vi "RG TAS v4.vi"() -> ()   [LabVIEW 2015]
uses:
  <vilib>/Analysis/2dsp.llb/Decimate (single shot, DBL).vi
  <vilib>/DAQmx/read.llb/DAQmx Read (Analog Wfm 1Chan NSamp).vi
  Chaz TAS - DR/Sub VIs/Mono/global_Test.vi
  <vilib>/Instr/_visa.llb/VISA Configure Serial Port (Instr).vi
  Sub VIs/global tas.vi
  <vilib>/DAQmx/miscellaneous.llb/DAQmx Fill In Error Info.vi
  <vilib>/Utility/file.llb/Write To Spreadsheet File (DBL).vi
  <vilib>/Waveform/WDTOps.llb/WDT Index Channel DBL.vi
  Program Files/National Instruments/LabVIEW 2014/instr.lib/Tektronix DPO MSO 2000 4000 Series/Tektronix DPO MSO 2000 4000 Series.lvlib
  <vilib>/Analysis/NI_AALPro.lvlib
panel:
  out "DAQ Loop":i32
  out "Scope Error Counter":i32
  out "Scope time axis":dbl[](array[numeric])
  in  "Stop acquisition":bool
  out "Grating":i32
  in  "2b - Spectrum":bool
  in  "2a - Kinetic":bool
  in  "Stop":bool
  out "Btrace Readout Counter":i32=2
  in  "Stop Btrace Measurement":bool
  out "Readout Counter":i32=2
  in  "Stop Measurement":bool
  in  "Calculate Output Method":T1(ring)
  in  "Parameters":T2(tab)
  in  "Shutter flow control":u16(ring) items=["None"=0, "XON/XOFF"=1, "RTS/CTS"=2, "DTR/DSR"=4]
  in  "Shutter stop bits":u16(ring)=10 items=["1.0"=10, "1.5"=15, "2.0"=20]
  in  "Shutter parity":u16(ring) items=["None", "Odd", "Even", "Mark", "Space"]
  in  "Shutter data bits":u16=8 min=5 max=8 step=1
  in  "Shutter VISA resource name":refnum<visa-resource-name>="COM1"
  in  "Shutter baud rate":u32=9600
  in  "Shutter open string":string="+100 10\n"
  in  "1 - Move Shutter":bool
  in  "3 - Move mono":bool
  out "Current wavelength (Oriel)":dbl format="%#_13g"
  in  "Monochromator Type":bool
  out "Start Wavelength":dbl min=0.0 format="%.3f"
  out "End Wavelength":dbl=100.0 min=0.0 format="%.3f"
  out "Interval Wavelength":dbl=10.0 min=0.0 format="%.3f"
  out "Current Wavelength (PTI)":dbl=300.0 min=300.0 max=2000.0 step=1.0
  in  "Is IR":bool caption="Grating"
  in  "Mono VISA name":refnum<visa-resource-name>
  in  "Mono 2 VISA name":refnum<visa-resource-name>
  out "DAQ dt":dbl=5e-06
  in  "DAQ End Time":dbl=0.05
  in  "DAQ rate":i32=1250000
  in  "DAQ Trigger Level (V)":dbl=0.2
  out "DAQ Number of Samples":dbl=10000.0
  in  "DAQ average number of points":dbl=1.0
  out "DAQ final number of points":dbl
  in  "DAQ Input Channel":tag="Dev1/ai0"
  in  "100% Reflectance Standard (V)":dbl=1.0
  in  "DAQ Card":enum16{"USB-6211", "USB-6251"}(ring)=enum."USB-6251"
  in  "DAQ Input Config":i32(ring)=10106 items=["default"=-1, "RSE"=10083, "NRSE"=10078, "Differential"=10106, "Pseudodifferential"=12529]
  in  "Record Length":u32(ring)=10 items=["1000 points"=1, "10k points"=10, "100k points"=100, "1M points"=1000, "5M points"=5000, "10M points"=10000]
  in  "Acquisition Type":u16(ring)=2 items=["Sample", "Peak Detect", "Hi Res", "Envelope", "Average"]
  in  "Scope average\nnumber of points":dbl=1.0
  in  "Averages on scope":i32=1
  in  "Using TDS Scope?":bool
  in  "CH2 Impedance":u16(ring) items=["1M", "75", "50"]
  in  "CH1 Impedance":u16(ring)=2 items=["1M", "75", "50"]
  in  "Scope VISA resource name":refnum<visa-resource-name>="USB0::0x0699::0x0410::C022077::INSTR"
  in  "Scope Timeout (ms)":u32=30000
  in  "Channel TAS (0: Channel 1)":u16(ring) caption="Channel TAS" items=["Channel 1", "Channel 2", "Channel 3", "Channel 4", "Math", "Reference A", "Reference B", "Reference C", "Reference D"]
  in  "Channel TPC (0: Channel 1)":u16(ring)=1 caption="Channel TPC" items=["Channel 1", "Channel 2", "Channel 3", "Channel 4", "Math", "Reference A", "Reference B", "Reference C", "Reference D"]
  in  "Scope Timebase":dbl=0.0004 format="%^#_3e"
  in  "Trigger Source":u16(ring)=1 items=["Channel 1", "Channel 2", "Channel 3", "Channel 4", "AC Line", "Aux", "Digital Channel 0", "Digital Channel 1", "Digital Channel 2", "Digital Channel 3", "Digital Channel 4", "Digital Channel 5", "Digital Channel 6", "Digital Channel 7", "Digital Channel 8", "Digital Channel 9", "Digital Channel 10", "Digital Channel 11", "Digital Channel 12", "Digital Channel 13", "Digital Channel 14", "Digital Channel 15", "RF"]
  out "Final number of\nscope points":dbl=10000.0
  in  "Vertical Coupling TAS (1: DC)":u16(ring)=1 caption="Vertical Coupling TAS" items=["AC", "DC", "Ground"]
  in  "Probe Attenuation TAS (10.0)":dbl=1.0 caption="Probe Attenuation TAS"
  in  "Bandwidth CHTAS (0: FULL)":i32(ring) caption="Bandwidth CH TAS" items=["FULL", "250 MHz", "150 MHz", "20 MHz"]
  in  "Vertical Offset CH TAS (0.0 divs)":dbl=0.4 caption="Vertical Offset CH TAS (in V)"
  in  "Vertical Range CH TAS (10.0 V)":dbl=0.2 caption="Vertical Range CH TAS"
  in  "Trigger Level (V)":dbl=0.25
  in  "Vertical Coupling TPC (1: DC)":u16(ring)=1 caption="Vertical Coupling TPC" items=["AC", "DC", "Ground"]
  in  "Probe Attenuation TPC (1.0)":dbl=1.0 caption="Probe Attenuation TPC"
  in  "Vertical Range TPC (10.0 V)":dbl=0.2 caption="Vertical Range TPC"
  in  "Bandwidth CH TPC (0: FULL)":i32(ring) caption="Bandwidth CH TPC" items=["FULL", "250 MHz", "150 MHz", "20 MHz"]
  in  "Vertical Offset CH TPC (0.0 divs)":dbl caption="Vertical Offset CH TPC (in V)"
  in  "TPC Multiplication factor":dbl=1.0
  out "Number of scope readouts":i32
  in  "Scope Channel Read":bool
  in  "LED on (s)":dbl
  in  "LED off (s)":dbl
  in  "PIA Mode":bool
  in  "LEDs (constant irrad.)":bool caption="LEDs"
  in  "DAQ LED line":string="Dev1/port1/line0"
  in  "Control LEDs?":bool
  out "Scope pretrigger points":dbl=1000.0
  out "Scope CH1 DOD data (A-B final)":waveform(dbl)(graph)
  out "Scope CH1 DOD data (A final)":waveform(dbl)(graph)={"t0"=timestamp(-4.0000000000040004e-05 s since 1904-01-01), "dt"=4.0000000000000003e-07, "Y"=array[10000 elements]}
  out "Scope CH2 data (final)":waveform(dbl)(graph)={"t0"=timestamp(-4.0000000000040004e-05 s since 1904-01-01), "dt"=4.0000000000000003e-07, "Y"=array[10000 elements]}
  out "DAQ DOD data (final)":waveform(dbl)(graph)={"t0"=timestamp(0 s since 1904-01-01), "dt"=5e-06, "Y"=array[10000 elements]}
  out "B trace (Channel1)":waveform(dbl)(graph)
  in  "Amplification Factor":dbl=400.0
  out "Background level (on Amp)":dbl=30.577247161746392
  out "Background level (V)":dbl=0.08993307988748939
  in  "Trace B ?":bool
  out "Folder Created":bool
  in  "Sample Name":string="Sample"
  in  "TAS2014  Path":path=path "D:/Solar Fuels Data" caption="Folder"
  out "Path to Files":path=path "D:/Solar Fuels Data/Sample"
  out "Scope Average Channel2":waveform(dbl)(graph)={"t0"=timestamp(-4.0000000000040004e-05 s since 1904-01-01), "dt"=4.0000000000000003e-07, "Y"=array[10000 elements]}
  out "Scope Average Channel1":waveform(dbl)(graph)={"t0"=timestamp(-4.0000000000040004e-05 s since 1904-01-01), "dt"=4.0000000000000003e-07, "Y"=array[10000 elements]}
  out "DAQ Average Data":waveform(dbl)(graph)={"t0"=timestamp(0 s since 1904-01-01), "dt"=5e-06, "Y"=array[10000 elements]}
  in  "Number of Averages":i32=2
  out "DAQ Live Data":waveform(dbl)(graph)={"t0"=timestamp(0 s since 1904-01-01), "dt"=4.999999999999959e-06, "Y"=array[10000 elements]}
  # "Acquisition"
  # "Format: +100\\s20\\n OR \\F3\\002\\C1"
  # "Set COM ports for PTI\nmonochromators. If there\nis only 1 monochromator\npresent, leave Mono 2\nVISA name empty."
  # "DAQ Controls"
  # "DAQ Indicators"
  # "(Max = 250k/1.25M for\n6211/6251 DAQ cards)"
  # "Default is differential (connected ports are 15 and 16 on DAQ card).\n* For CH-TAS, input config should be RSE."
  # "Recommended Parameters for Different Scope Models"
  # "DPO3012"
  # "Record Length = 10k\nScope average number of points = 1"
  # "Acquisition Type = Hi Res\nAverages on scope = 1"
  # "DPO2012B"
  # "Record Length = 1M\nScope average number of points = 100"
  # "Acquisition Type = Average\nAverages on scope = 4"
  # "TDS3012C"
  # "Record Length = 10k\nScope average number of points = 1"
  # "Acquisition Type = Sample\nAverages on scope = 1"
  # "Channel 1"
  # "Channel 2"
  # "* For DPO2012B, impedance must be 1M for both channels!"
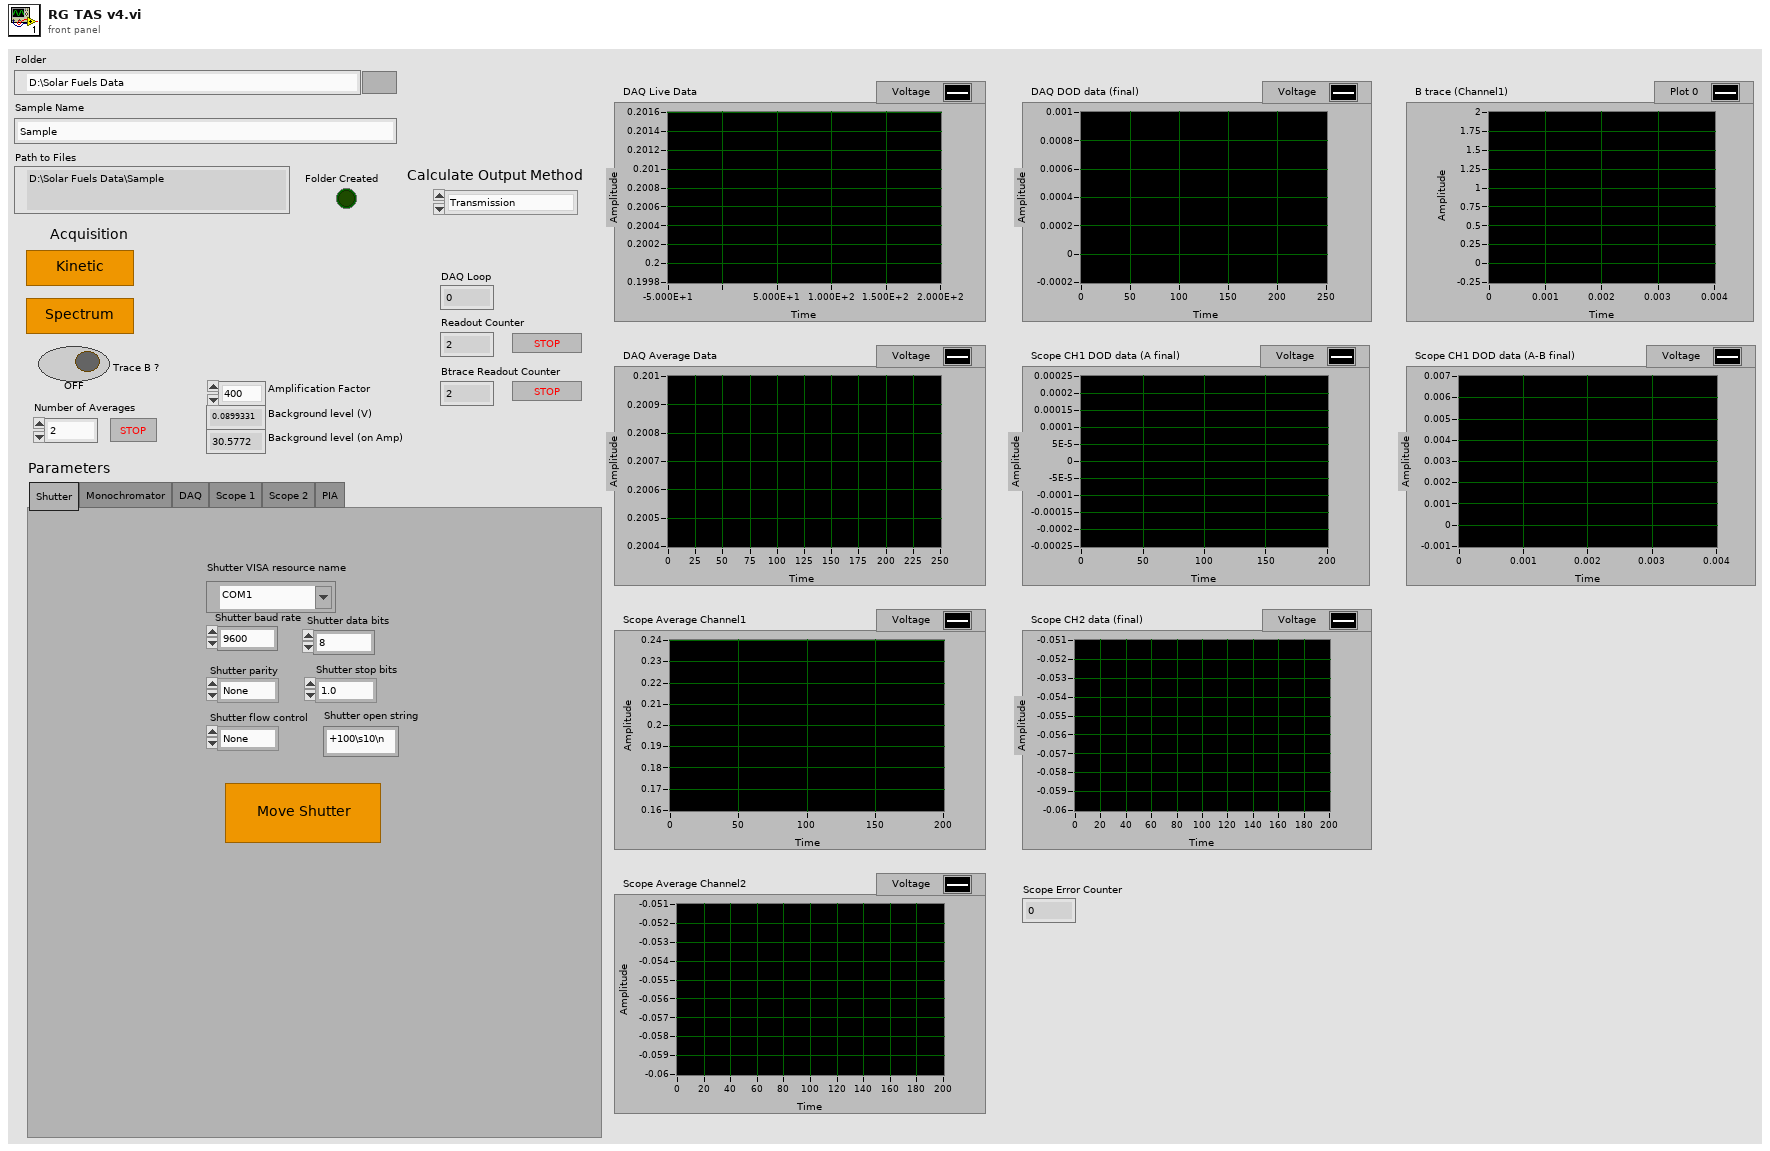
[diagram p1: front panel]
types:
  T1 = enum16{"Transmission", "Reflectance", "Kubelka-Munk"}
  T2 = enum32{"Shutter", "Monochromator", "DAQ", "Scope 1", "Scope 2", "PIA"}
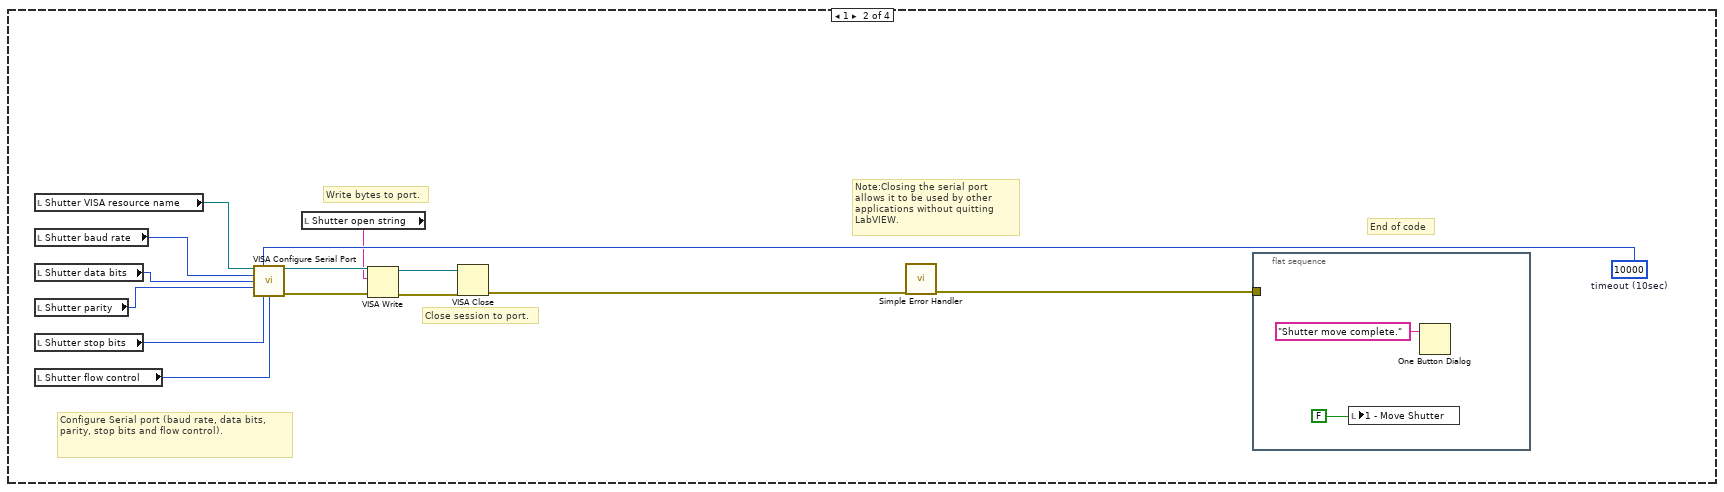
[diagram p4: hidden frame]
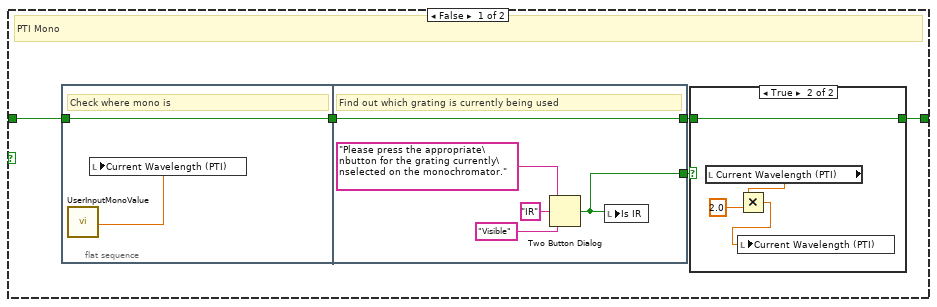
[diagram p5: hidden frame]
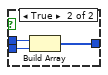
[diagram p8: hidden frame]
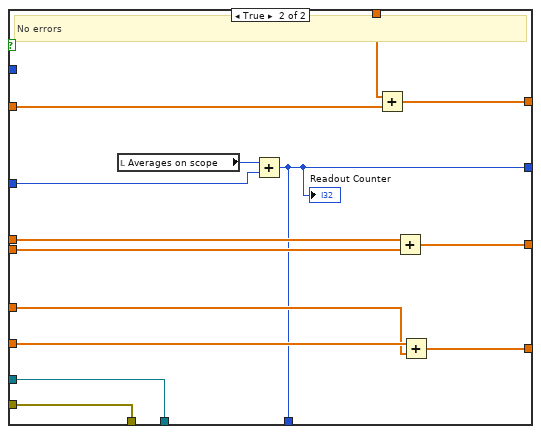
[diagram p9: hidden frame]
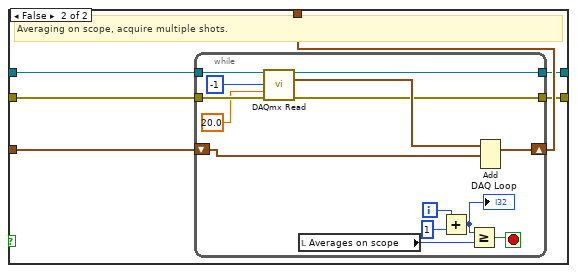
[diagram p11: hidden frame]
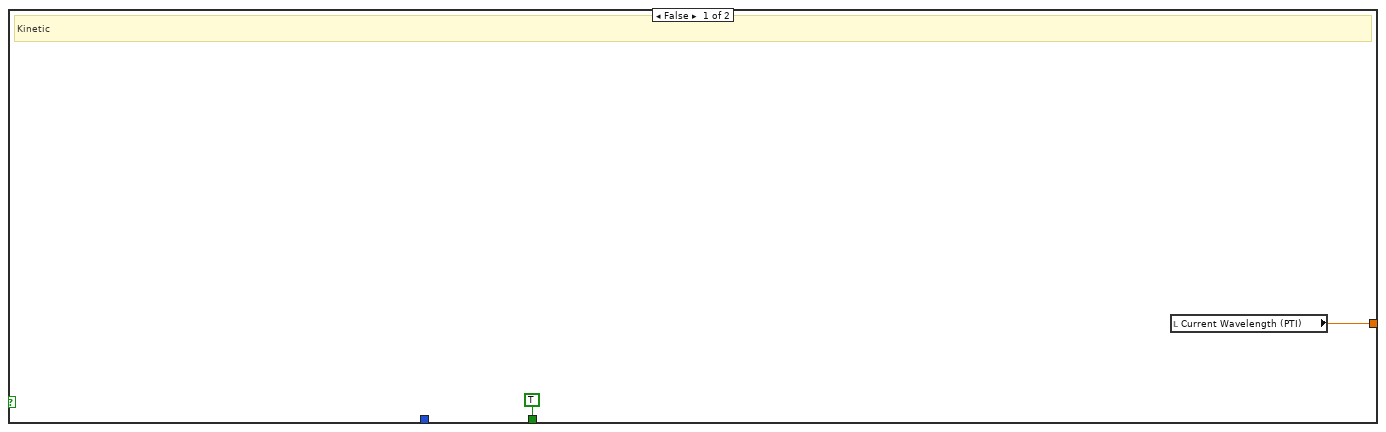
[diagram p12: hidden frame]
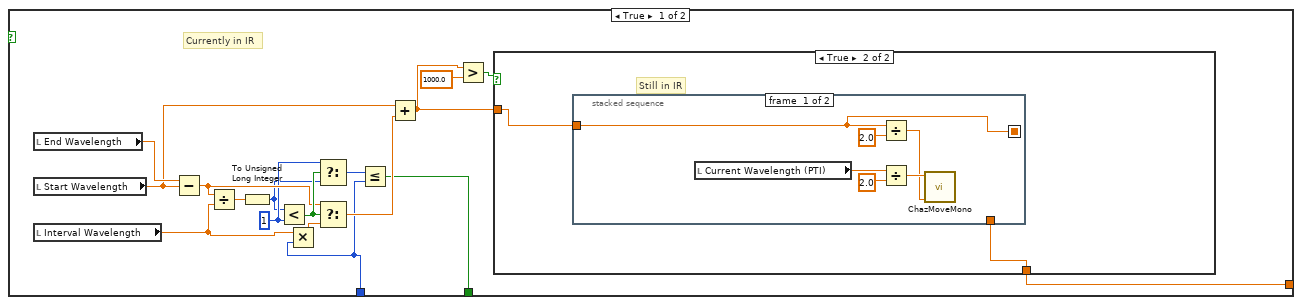
[diagram p13: hidden frame]
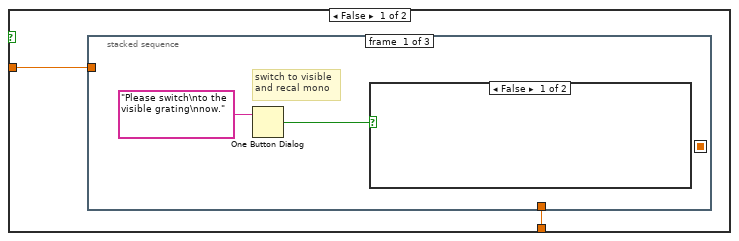
[diagram p14: hidden frame]
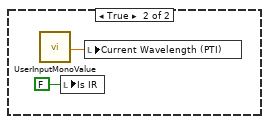
[diagram p15: hidden frame]
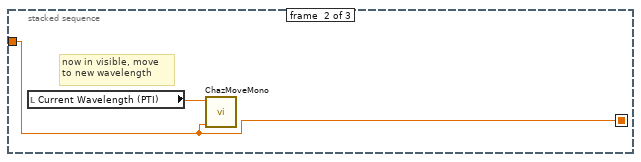
[diagram p16: hidden frame]
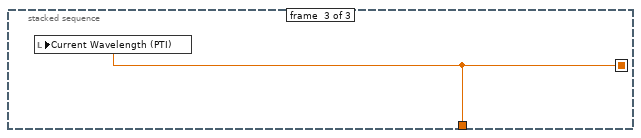
[diagram p17: hidden frame]
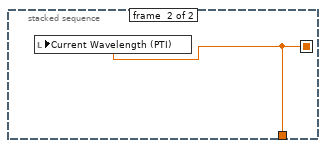
[diagram p18: hidden frame]
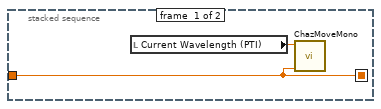
[diagram p19: hidden frame]
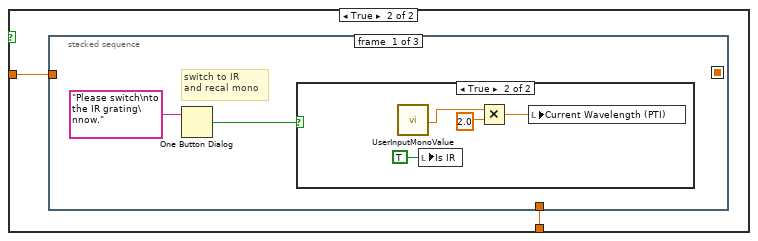
[diagram p20: hidden frame]
diagram:
  n1 = while {
    stop <- "Stop" stop-if-true
    # "True = Oriel"
    n2 = Or(x="2a - Kinetic", y="2b - Spectrum") -> (x .or. y?=w6:bool)
    n3 = Build Array(FALSE, "1 - Move Shutter", w6, "3 - Move mono") -> (w11:bool[])
    n4 = Search 1D Array(1D array=w11, element=TRUE) -> (index of element=w4:i32)  [unwired: 1 in]
    n5 = flat-sequence {
      tunnel: w4 -> [w37]
      tunnel: [w37] -> w3
      tunnel: "Monochromator Type" -> [w15]
      tunnel: [w15] -> w1
      frame #0 {
        # "Calculate DAQ parameters"
        # "Calculate Scope Parameters"
        n6 = case shown="True" "Control LEDs?" {
          frame False {
          }
          frame True {
            n7 = call "RG DAQ control for PIA.vi"("lines"="DAQ LED line", "Initial value"="LEDs (constant irrad.)") -> ()  [unwired: 10 in]
          }
        }
        n8 = Multiply(x="DAQ End Time", y=1.1) -> (x*y=w16:dbl)
        n9 = Multiply(x="Record Length", y=u32 1000) -> (x*y=w25:u32)
        n10 = Multiply(x="DAQ rate", y=w16) -> (x*y=w24:dbl)
        "DAQ Number of Samples" <- w24
        n11 = Reciprocal(x="DAQ rate") -> (1/x=→"DAQ dt":dbl)
        n12 = Divide(x="Number of Averages", y="Averages on scope") -> (x/y=→"Number of scope readouts":dbl)
        n13 = Divide(x=w25, y="Scope average\nnumber of points") -> (x/y=w29:dbl)
        "Final number of\nscope points" <- w29
        n14 = Divide(x=w29, y=10.0) -> (x/y=→"Scope pretrigger points":dbl)
        n15 = Wait (ms)(milliseconds to wait=u32 1000) -> ()  [unwired: 1 out]
        n16 = Divide(x=w24, y="DAQ average number of points") -> (x/y=→"DAQ final number of points":dbl)
        n17 = global write "global_Test.vi" "Mono VISA name"("Mono VISA name") -> ()
        n18 = global write "global_Test.vi" "Mono 2 VISA name"("Mono 2 VISA name") -> ()
      }
    }
    n19 = case shown="2" w3 {
      tunnel: w1 -> [_ _ w56 w966]
      frame 0, Default {
      }
      frame 1 {
        w48 = u32 10000  # timeout (10sec)
        # "End of code"
        # "Note:Closing the serial port allows it to be used by other applications without quitting LabVIEW."
        # "Close session to port."
        # "Configure Serial port (baud rate, data bits, parity, stop bits and flow control)."
        # "Write bytes to port."
        n20 = local read "Shutter VISA resource name"() -> (w47:refnum<visa-resource-name>)
        n21 = local read "Shutter baud rate"() -> (w46:u32)
        n22 = local read "Shutter data bits"() -> (w45:u16)
        n23 = local read "Shutter parity"() -> (w44:u16)
        n24 = local read "Shutter stop bits"() -> (w43:u16)
        n25 = local read "Shutter flow control"() -> (w42:u16)
        n26 = call-poly "VISA Configure Serial Port"("VISA resource name"=w47, "timeout (10sec)"=w48, "baud rate (9600)"=w46, "data bits (8)"=w45, "parity (0:none)"=w44, "stop bits (10: 1 bit)"=w43, "flow control (0:none)"=w42) -> ("VISA resource name out"=w49:refnum<visa-resource-name>, "error out"=w50:errorcluster)  [unwired: 2 in, 5 out]
        n27 = local read "Shutter open string"() -> (w41:string)
        n28 = VISA Write(VISA resource name=w49, write buffer=w41, error in (no error)=w50) -> (VISA resource name out=w52:refnum<visa-resource-name>, error out=w53:errorcluster)  [unwired: 1 out]
        n29 = VISA Close(VISA resource name=w52, error in (no error)=w53) -> (error out=w51:errorcluster)
        n30 = call <vilib>:"Simple Error Handler.vi"("error in (no error)"=w51) -> ("error out"=w40:errorcluster)  [unwired: 1 in, 7 out]
        n31 = flat-sequence {
          tunnel: w40 -> [_]
          frame #0 {
            n32 = local write "1 - Move Shutter"(FALSE ("Move Shutter")) -> ()
            n33 = One Button Dialog(message="Shutter move complete.") -> ()  [unwired: 1 in, 1 out]
          }
        }
      }
      frame 2 {
        n34 = Build Path(base path="TAS2014  Path", name or relative path="Sample Name") -> (appended path=w67:path)
        n35 = call <vilib>:"Check if File or Folder Exists.vi"("path"=w67) -> ("file or folder exists?"=w66:bool, "dup path"=w65:path)  [unwired: 8 in, 1 out]
        n36 = case shown="False" w66 {
          tunnel: w65 -> [w958 w964]
          tunnel: [w957 w964] -> w60
          frame False {
            n37 = Create Folder(path (use dialog)=w958) -> (created path=w957:path)  [unwired: 2 in, 2 out]
            n38 = local write "Folder Created"(TRUE ("Folder Created")) -> ()
          }
          frame True {
            n39 = Two Button Dialog(message="Caution - folder already exists. Continue to overwrite data?", 1:"Yes, go for it!" ("F button name (\"Cancel\")"), 2:"No, help me!" ("T button name (\"OK\")")) -> (T button?=w959:bool)
            n40 = local write "Folder Created"(FALSE ("Folder Created")) -> ()
            n41 = Stop(stop? (T)=w959) -> ()
          }
        }
        "Path to Files" <- w60
        n42 = case shown="True" w56 {
          tunnel: w56 -> [w71 w86]
          tunnel: [w69 w85] -> w57
          frame False {
            # "PTI Mono"
            n43 = flat-sequence {
              tunnel: [w78] -> w72
              tunnel: w71 -> [w78]
              tunnel: w72 -> [w84]
              tunnel: [w84] -> w70
              tunnel: [w80] -> w68
              frame #0 {
                # "Check where mono is"
                n44 = call "UserInputMonoValue.vi"() -> ("Monochromator readout"=w79:dbl)  [unwired: 17 in, 2 out]
                n45 = local write "Current Wavelength (PTI)"(w79) -> ()
              }
              frame #1 {
                # "Find out which grating is currently being used"
                n46 = Two Button Dialog(message="Please press the appropriate\nbutton for the grating currently\nselected on the monochromator.", 1:"Visible" ("F button name (\"Cancel\")"), 2:"IR" ("T button name (\"OK\")")) -> (T button?=w80:bool)
                n47 = local write "Is IR"(w80) -> ()
              }
            }
            n48 = case shown="True" w68 {
              tunnel: w70 -> [w73 w77]
              tunnel: [w73 w77] -> w69
              frame False {
              }
              frame True {
                n49 = local read "Current Wavelength (PTI)"() -> (w75:dbl)
                n50 = Multiply(x=w75, y=2.0) -> (x*y=w74:dbl)
                n51 = local write "Current Wavelength (PTI)"(w74) -> ()
              }
            }
          }
          frame True {
            # "Oriel Mono"
            n52 = flat-sequence {
              tunnel: w86 -> [w90]
              tunnel: [w90] -> w85
              frame #0 {
                n53 = call "m_open.vi"() -> ("error out"=w91:errorcluster, "configuration file path copy"=w87:path)  [unwired: 2 in]
                n54 = call "GetWave.vi"("error in (no error)"=w91) -> ("error out"=w89:errorcluster, "Present Wavelength"=w88:dbl)  [unwired: 1 in]
                n55 = call "m_close.vi"("error in (no error)"=w89, "configuration file path"=w87) -> ()  [unwired: 2 out]
                n56 = local write "Current wavelength (Oriel)"(w88) -> ()
              }
            }
          }
        }
        n57 = local read "2b - Spectrum"() -> (w62:bool)
        n58 = global write "global tas.vi" "Root Path"(w60) -> ()
        n59 = case shown="True" w62 {
          tunnel: w60 -> [w95 w96]
          tunnel: [w95 w96] -> w58
          frame False {
          }
          frame True {
            n60 = call "RG Get Spectrum Wavelengths.vi"() -> ("Wavelength interval"=→"Interval Wavelength":i32, "End wavelength"=→"End Wavelength":i32, "Start wavelength"=→"Start Wavelength":i32)  [unwired: 9 in]
          }
        }
        n61 = flat-sequence {
          tunnel: [w92] -> w59
          tunnel: w58 -> [_]
          frame #0 {
            n62 = call "Prompt User for Input"() -> ("yes"=w92:bool)  [unwired: 18 in, 1 out]
          }
        }
        n63 = while {
          tunnel: [w177] -> w61
          tunnel: w59 -> [w172]
          tunnel: w57 -> [w165]
          i -> [w166]
          stop <- w196 stop-if-true
          w257 = TRUE  # Reset (True)
          w131 = 0
          w260 = FALSE  # ID Query (True)
          w293 = FALSE  # Enable Continuous Acquisition Mode (True)
          # "Scope t0"
          # "Scope dt"
          # "DAQ index to make\nsure DAQ acquisition\nis finished before\ndoing B trace."
          # "Scope time\naxis"
          # "Scope time axis"
          # "Current wavelength"
          # "Current Wavelength"
          # "Make sure the 20s is waited before starting to acquire the data if shutter moves."
          # "Set time so that trigger\nis at t = 0"
          # "Get pre laser light level"
          # "Change cases for old TDS scope models because of differences in programming commands."
          # "Get pre laser light level (V) for DAQ and Scope"
          # "Disable time delay"
          # "Configure Timebase"
          # "Disable continous acquisition"
          # "Configure Trigger"
          # "If reading 2 channels, combine Channel A\n and Channel B so that both channels are read"
          # "Configure Channel B"
          # "Configure Channel A"
          # "Check the initial position of the shutter, and move if Doing Trace B and Spectrum"
          n64 = local read "2b - Spectrum"() -> (w169:bool)
          n65 = case shown="False" w165 {
            tunnel: [w518 w609] -> w195
            tunnel: [w515 w608] -> w193
            tunnel: [w517 w607] -> w176
            tunnel: w169 -> [w519 w606]
            tunnel: w166 -> [w520 w605]
            frame False {
              # "PTI Monochromator"
              n66 = flat-sequence {
                tunnel: w520 -> [w524]
                tunnel: w519 -> [w523]
                tunnel: [w522] -> w518
                tunnel: [w521] -> w516
                tunnel: [w604] -> w517
                tunnel: w516 -> [w604]
                tunnel: [w603] -> w515
                frame #0 {
                  n67 = case shown="True" w523 {
                    tunnel: w524 -> [_ w529]
                    tunnel: [TRUE w528] -> w522
                    tunnel: [w526 w527] -> w521
                    frame False {
                      # "Kinetic"
                      n68 = local read "Current Wavelength (PTI)"() -> (w526:dbl)
                    }
                    frame True {
                      # "Spectrum"
                      n69 = case shown="False" "Is IR" {
                        tunnel: w529 -> [w533 w569]
                        tunnel: [w534 w568] -> w528
                        tunnel: [w532 w567] -> w527
                        frame True {
                          w542 = u32 1 ("y")
                          # "Currently in IR"
                          n70 = local read "End Wavelength"() -> (w540:dbl)
                          n71 = local read "Start Wavelength"() -> (w538:dbl)
                          n72 = local read "Interval Wavelength"() -> (w535:dbl)
                          n73 = Subtract(x=w540, y=w538) -> (x-y=w543:dbl)
                          n74 = Divide(x=w543, y=w535) -> (x/y=w545:dbl)
                          n75 = To Unsigned Long Integer(number=w545) -> (unsigned 32bit integer=w541:u32)
                          n76 = Less?(x=w541, y=w542) -> (x < y?=w544:bool)
                          n77 = Multiply(x=w535, y=w533) -> (x*y=w536:dbl)
                          n78 = Select(t=w542, s=w544, f=w541) -> (s? t:f=w539:u32)
                          n79 = Select(t=w543, s=w544, f=w536) -> (s? t:f=w537:dbl)
                          n80 = Less Or Equal?(x=w539, y=w533) -> (x <= y?=w534:bool)
                          n81 = Add(x=w538, y=w537) -> (x+y=w531:dbl)
                          n82 = Greater?(x=w531, y=1000.0) -> (0:w546:bool)
                          n83 = case shown="True" w546 {
                            tunnel: [w549 w558] -> w532
                            tunnel: w531 -> [w548 w557]
                            frame False {
                              n84 = stacked-sequence {
                                seq-local: [_ w554 _] -> [_ _ w556]
                                tunnel: [_ _ w556] -> w549
                                tunnel: w548 -> [_ w554 _]
                                frame #0 {
                                # "switch to visible\nand recal mono"
                                n85 = One Button Dialog(message="Please switch\nto the visible grating\nnow.") -> (true=w550:bool)  [unwired: 1 in]
                                n86 = case shown="False" w550 {
                                frame False {
                                }
                                frame True {
                                n87 = call "UserInputMonoValue.vi"() -> ("Monochromator readout"=w552:dbl)  [unwired: 17 in, 2 out]
                                n88 = local write "Is IR"(FALSE ("Is IR")) -> ()
                                n89 = local write "Current Wavelength (PTI)"(w552) -> ()
                                }
                                }
                                }
                                frame #1 {
                                # "now in visible, move \nto new wavelength"
                                n90 = local read "Current Wavelength (PTI)"() -> (w555:dbl)
                                n91 = call "ChazMoveMono.vi"("Move to"=w554, "Current"=w555) -> ()  [unwired: 8 in, 2 out]
                                }
                                frame #2 {
                                n92 = local write "Current Wavelength (PTI)"(w556) -> ()
                                }
                              }
                            }
                            frame True {
                              # "Still in IR"
                              n93 = stacked-sequence {
                                seq-local: [w559 _] -> [_ w565]
                                tunnel: [_ w565] -> w558
                                tunnel: w557 -> [w559 _]
                                frame #0 {
                                n94 = local read "Current Wavelength (PTI)"() -> (w564:dbl)
                                n95 = Divide(x=w559, y=2.0) -> (x/y=w560:dbl)
                                n96 = Divide(x=w564, y=2.0) -> (x/y=w561:dbl)
                                n97 = call "ChazMoveMono.vi"("Move to"=w560, "Current"=w561) -> ()  [unwired: 8 in, 2 out]
                                }
                                frame #1 {
                                n98 = local write "Current Wavelength (PTI)"(w565) -> ()
                                }
                              }
                            }
                          }
                        }
                        frame False {
                          w577 = u32 1 ("y")
                          # "Currently in Visible"
                          n99 = local read "End Wavelength"() -> (w575:dbl)
                          n100 = local read "Start Wavelength"() -> (w573:dbl)
                          n101 = local read "Interval Wavelength"() -> (w570:dbl)
                          n102 = Subtract(x=w575, y=w573) -> (x-y=w578:dbl)
                          n103 = Divide(x=w578, y=w570) -> (x/y=w580:dbl)
                          n104 = To Unsigned Long Integer(number=w580) -> (unsigned 32bit integer=w576:u32)
                          n105 = Less?(x=w576, y=w577) -> (x < y?=w579:bool)
                          n106 = Multiply(x=w570, y=w569) -> (x*y=w571:dbl)
                          n107 = Select(t=w577, s=w579, f=w576) -> (s? t:f=w574:u32)
                          n108 = Select(t=w578, s=w579, f=w571) -> (s? t:f=w572:dbl)
                          n109 = Less Or Equal?(x=w574, y=w569) -> (x <= y?=w568:bool)
                          n110 = Add(x=w573, y=w572) -> (x+y=w566:dbl)
                          n111 = Greater?(x=w566, y=1000.0) -> (0:w581:bool)
                          n112 = case shown="False" w581 {
                            tunnel: [w584 w589] -> w567
                            tunnel: w566 -> [w583 w588]
                            frame False {
                              # "Still in Visible"
                              n113 = stacked-sequence {
                                seq-local: [w585 _] -> [_ w587]
                                tunnel: [_ w587] -> w584
                                tunnel: w583 -> [w585 _]
                                frame #0 {
                                n114 = local read "Current Wavelength (PTI)"() -> (w586:dbl)
                                n115 = call "ChazMoveMono.vi"("Move to"=w585, "Current"=w586) -> ()  [unwired: 8 in, 2 out]
                                }
                                frame #1 {
                                n116 = local write "Current Wavelength (PTI)"(w587) -> ()
                                }
                              }
                            }
                            frame True {
                              n117 = stacked-sequence {
                                seq-local: [_ w596 _] -> [_ _ w602]
                                tunnel: [_ _ w602] -> w589
                                tunnel: w588 -> [_ w596 _]
                                frame #0 {
                                # "switch to IR\nand recal mono"
                                n118 = One Button Dialog(message="Please switch\nto the IR grating\nnow.") -> (true=w590:bool)  [unwired: 1 in]
                                n119 = case shown="True" w590 {
                                frame False {
                                }
                                frame True {
                                n120 = call "UserInputMonoValue.vi"() -> ("Monochromator readout"=w594:dbl)  [unwired: 17 in, 2 out]
                                n121 = local write "Is IR"(TRUE ("Is IR")) -> ()
                                n122 = Multiply(x=w594, y=2.0) -> (x*y=w592:dbl)
                                n123 = local write "Current Wavelength (PTI)"(w592) -> ()
                                }
                                }
                                }
                                frame #1 {
                                # "now in IR, move \nto new wavelength"
                                n124 = local read "Current Wavelength (PTI)"() -> (w599:dbl)
                                n125 = Divide(x=w596, y=2.0) -> (x/y=w597:dbl)
                                n126 = Divide(x=w599, y=2.0) -> (x/y=w598:dbl)
                                n127 = call "ChazMoveMono.vi"("Move to"=w597, "Current"=w598) -> ()  [unwired: 8 in, 2 out]
                                }
                                frame #2 {
                                n128 = local write "Current Wavelength (PTI)"(w602) -> ()
                                }
                              }
                            }
                          }
                        }
                      }
                    }
                  }
                }
                frame #1 {
                  n129 = call <vilib>:"General Error Handler.vi"() -> ("error out"=w603:errorcluster)  [unwired: 11 in, 4 out]
                }
              }
            }
            frame True {
              # "Oriel Monochromator"
              n130 = case shown="False" w606 {
                tunnel: [TRUE w639] -> w609
                tunnel: w605 -> [_ w626]
                tunnel: [w611 w624] -> w608
                tunnel: [w610 w623] -> w607
                frame False {
                  # "B trace OFF"
                  n131 = call "m_open.vi"() -> ("error out"=w613:errorcluster, "configuration file path copy"=w612:path)  [unwired: 2 in]
                  n132 = call "GetWave.vi"("error in (no error)"=w613) -> ("error out"=w621:errorcluster, "Present Wavelength"=w610:dbl)  [unwired: 1 in]
                  "Current wavelength (Oriel)" <- w610
                  n133 = Less Or Equal?(x=w610, y=590.0) -> (x <= y?=w620:bool)
                  n134 = Select(t=1.0, s=w620, f=2.0) -> (s? t:f=w617:dbl)
                  n135 = call "setgrat.vi"("error in (no error)"=w621, "Grating"=w617) -> ("error out"=w618:errorcluster)  [unwired: 1 in]
                  n136 = call "gowave.vi"("error in (no error)"=w618, "Destination Wavelength"=w610) -> ("error out"=w619:errorcluster)
                  n137 = call "m_close.vi"("error in (no error)"=w619, "configuration file path"=w612) -> ("error out"=w611:errorcluster)  [unwired: 1 out]
                }
                frame True {
                  w643 = u32 1 ("y")
                  # "B trace ON"
                  n138 = local read "End Wavelength"() -> (w641:dbl)
                  n139 = local read "Start Wavelength"() -> (w630:dbl)
                  n140 = local read "Interval Wavelength"() -> (w627:dbl)
                  n141 = Subtract(x=w641, y=w630) -> (x-y=w644:dbl)
                  n142 = Divide(x=w644, y=w627) -> (x/y=w646:dbl)
                  n143 = To Unsigned Long Integer(number=w646) -> (unsigned 32bit integer=w642:u32)
                  n144 = Less?(x=w642, y=w643) -> (x < y?=w645:bool)
                  n145 = Multiply(x=w627, y=w626) -> (x*y=w628:dbl)
                  n146 = Select(t=w643, s=w645, f=w642) -> (s? t:f=w640:u32)
                  n147 = Select(t=w644, s=w645, f=w628) -> (s? t:f=w629:dbl)
                  n148 = Less Or Equal?(x=w640, y=w626) -> (x <= y?=w639:bool)
                  n149 = Add(x=w630, y=w629) -> (x+y=w623:dbl)
                  n150 = call "m_open.vi"() -> ("error out"=w625:errorcluster, "configuration file path copy"=w638:path)  [unwired: 2 in]
                  n151 = Less Or Equal?(x=w623, y=590.0) -> (x <= y?=w631:bool)
                  n152 = local write "Current wavelength (Oriel)"(w623) -> ()
                  n153 = Select(t=1.0, s=w631, f=2.0) -> (s? t:f=w634:dbl)
                  n154 = call "setgrat.vi"("error in (no error)"=w625, "Grating"=w634) -> ("error out"=w633:errorcluster)  [unwired: 1 in]
                  n155 = call "gowave.vi"("error in (no error)"=w633, "Destination Wavelength"=w623) -> ("error out"=w632:errorcluster)
                  n156 = call "m_close.vi"("error in (no error)"=w632, "configuration file path"=w638) -> ("error out"=w624:errorcluster)  [unwired: 1 out]
                }
              }
            }
          }
          n157 = local read "Scope VISA resource name"() -> (w303:refnum<visa-resource-name>)
          n158 = local read "Trace B ?"() -> (w170:bool)
          n159 = And(x=w170, y=w169) -> (x .and. y?=w168:bool)
          n160 = Not Equal To 0?(x=w166) -> (x != 0?=w167:bool)
          n161 = And(x=w168, y=w167) -> (x .and. y?=w171:bool)
          n162 = Or(x=w172, y=w171) -> (x .or. y?=w173:bool)
          n163 = call "Initialize.vi"("error in (no error)"=w193, "Reset (True)"=w257, "ID Query (True)"=w260, "VISA resource name"=w303) -> ("error out"=w295:errorcluster, "VISA resource name out"=w294:refnum<visa-resource-name>)  [unwired: 6 in]
          n164 = local read "Scope Timeout (ms)"() -> (w125:u32)
          n165 = case shown="True" w173 {
            tunnel: [u32 0 ("millisecond timer value") w941] -> w110
            frame False {
            }
            frame True {
              w951 = u32 10000  # timeout (10sec)
              # "Note:Closing the serial port allows it to be used by other applications without quitting LabVIEW."
              # "Close session to port."
              # "Configure Serial port (baud rate, data bits, parity, stop bits and flow control)."
              # "Write bytes to port."
              n166 = call-poly "VISA Configure Serial Port"("VISA resource name"="Shutter VISA resource name", "timeout (10sec)"=w951, "baud rate (9600)"="Shutter baud rate", "data bits (8)"="Shutter data bits", "parity (0:none)"="Shutter parity", "stop bits (10: 1 bit)"="Shutter stop bits", "flow control (0:none)"="Shutter flow control") -> ("VISA resource name out"=w947:refnum<visa-resource-name>, "error out"=w946:errorcluster)  [unwired: 2 in, 5 out]
              n167 = VISA Write(VISA resource name=w947, write buffer="Shutter open string", error in (no error)=w946) -> (VISA resource name out=w944:refnum<visa-resource-name>, error out=w943:errorcluster)  [unwired: 1 out]
              n168 = VISA Close(VISA resource name=w944, error in (no error)=w943) -> (error out=w945:errorcluster)
              n169 = call <vilib>:"Simple Error Handler.vi"("error in (no error)"=w945) -> ()  [unwired: 1 in, 8 out]
              n170 = Wait (ms)(milliseconds to wait=u32 20000) -> (millisecond timer value=w941:u32)
            }
          }
          n171 = call "Configure Continuous Acquisition.vi"("error in (no error)"=w295, "Enable Continuous Acquisition Mode (T: Enable)"=w293, "VISA resource name"=w294) -> ("error out"=w129:errorcluster, "VISA resource name out"=w130:refnum<visa-resource-name>)  [unwired: 7 in]
          n172 = local read "Vertical Range CH TAS (10.0 V)"() -> (w288:dbl)
          n173 = local read "Vertical Offset CH TAS (0.0 divs)"() -> (w305:dbl)
          n174 = property class="Instr"(reference=w130, error in=w129, "General Settings:Timeout Value"=w125) -> (reference out=w128:refnum<visa-resource-name>, error out=w127:errorcluster)
          n175 = local read "Vertical Coupling TAS (1: DC)"() -> (w286:u16)
          n176 = local read "Bandwidth CHTAS (0: FULL)"() -> (w284:i32)
          n177 = local read "Probe Attenuation TAS (10.0)"() -> (w304:dbl)
          n178 = local read "Channel TAS (0: Channel 1)"() -> (w285:u16)
          n179 = Or(x=w195, y="Stop acquisition") -> (x .or. y?=w196:bool)
          n180 = local read "Vertical Offset CH TPC (0.0 divs)"() -> (w302:dbl)
          n181 = local read "Vertical Coupling TPC (1: DC)"() -> (w282:u16)
          n182 = local read "Probe Attenuation TPC (1.0)"() -> (w301:dbl)
          n183 = local read "Channel TPC (0: Channel 1)"() -> (w283:u16)
          n184 = local read "Vertical Range TPC (10.0 V)"() -> (w287:dbl)
          n185 = local read "Bandwidth CH TPC (0: FULL)"() -> (w281:i32)
          n186 = local read "Scope Timebase"() -> (w108:dbl)
          n187 = local read "Record Length"() -> (w278:u32)
          n188 = case shown="False" "Using TDS Scope?" {
            tunnel: w305 -> [w911 w939]
            tunnel: w304 -> [w910 w938]
            tunnel: w302 -> [w909 w937]
            tunnel: w301 -> [w908 w936]
            tunnel: w127 -> [w907 w935]
            tunnel: w128 -> [w906 w934]
            tunnel: w288 -> [w903 w931]
            tunnel: w287 -> [w902 w930]
            tunnel: w286 -> [w899 w927]
            tunnel: w285 -> [w898 w926]
            tunnel: w284 -> [w897 w925]
            tunnel: w283 -> [w896 w924]
            tunnel: w282 -> [w895 w923]
            tunnel: w281 -> [w894 w922]
            tunnel: w278 -> [w893 w921]
            tunnel: [w891 w919] -> w277
            tunnel: [w889 w917] -> w276
            tunnel: "CH1 Impedance" -> [w887 w915]
            tunnel: "CH2 Impedance" -> [w886 w914]
            tunnel: w108 -> [w885 w913]
            tunnel: 10.0 ("Position (10 %)") -> [w884 w912]
            frame True {
              n189 = call "RG Configure Channel TDS3012C.vi"("VISA resource name"=w906, "Input Impedance (0: 1M ohm)"=w887, "Channel (0: Channel 1)"=w898, "Vertical Coupling (1: DC)"=w899, "Probe Attenuation (1)"=w910, "error in (no error)"=w907, "Vertical Range (10.0 V)"=w903, "Vertical Offset (0.0 V)"=w911, "Bandwidth (0: FULL)"=w897) -> ("VISA resource name out"=w905:refnum<visa-resource-name>, "error out"=w904:errorcluster)  [unwired: 5 in]
              n190 = call "RG Configure Channel TDS3012C.vi"("VISA resource name"=w905, "Input Impedance (0: 1M ohm)"=w886, "Channel (0: Channel 1)"=w896, "Vertical Coupling (1: DC)"=w895, "Probe Attenuation (1)"=w908, "error in (no error)"=w904, "Vertical Range (10.0 V)"=w902, "Vertical Offset (0.0 V)"=w909, "Bandwidth (0: FULL)"=w894) -> ("VISA resource name out"=w900:refnum<visa-resource-name>, "error out"=w901:errorcluster)  [unwired: 5 in]
              n191 = call "RG Configure Timebase TDS3012C.vi"("Record Length (10: 10k points)"=w893, "error in (no error)"=w901, "Position (10 %)"=w884, "Timebase (0.0005 s)"=w885, "VISA resource name"=w900) -> ("error out"=w890:errorcluster, "VISA resource name out"=w892:refnum<visa-resource-name>)  [unwired: 5 in]
              n192 = call "RG Configure Delay TDS3012C.vi"("error in (no error)"=w890, "Enable Delay (T: Enable)"=FALSE, "VISA resource name"=w892) -> ("error out"=w889:errorcluster, "VISA resource name out"=w891:refnum<visa-resource-name>)  [unwired: 7 in]
            }
            frame False {
              n193 = call "Configure Channel.vi"("VISA resource name"=w934, "Input Impedance (0: 1M ohm)"=w915, "Channel (0: Channel 1)"=w926, "Vertical Coupling (1: DC)"=w927, "Probe Attenuation (1)"=w938, "error in (no error)"=w935, "Vertical Range (10.0 V)"=w931, "Vertical Offset (0.0 V)"=w939, "Bandwidth (0: FULL)"=w925) -> ("VISA resource name out"=w933:refnum<visa-resource-name>, "error out"=w932:errorcluster)  [unwired: 5 in]
              n194 = call "Configure Channel.vi"("VISA resource name"=w933, "Input Impedance (0: 1M ohm)"=w914, "Channel (0: Channel 1)"=w924, "Vertical Coupling (1: DC)"=w923, "Probe Attenuation (1)"=w936, "error in (no error)"=w932, "Vertical Range (10.0 V)"=w930, "Vertical Offset (0.0 V)"=w937, "Bandwidth (0: FULL)"=w922) -> ("VISA resource name out"=w928:refnum<visa-resource-name>, "error out"=w929:errorcluster)  [unwired: 5 in]
              n195 = call "Configure Timebase.vi"("Record Length (10: 10k points)"=w921, "error in (no error)"=w929, "Position (10 %)"=w912, "Timebase (0.0005 s)"=w913, "VISA resource name"=w928) -> ("error out"=w918:errorcluster, "VISA resource name out"=w920:refnum<visa-resource-name>)  [unwired: 5 in]
              n196 = call "Configure Delay.vi"("error in (no error)"=w918, "Enable Delay (T: Enable)"=FALSE, "VISA resource name"=w920) -> ("error out"=w917:errorcluster, "VISA resource name out"=w919:refnum<visa-resource-name>)  [unwired: 7 in]
            }
          }
          n197 = Multiply(x=w108, y=1800.0) -> (x*y=w106:dbl)
          n198 = flat-sequence {
            tunnel: [w313] -> w124
            tunnel: [w312] -> w123
            tunnel: [w311] -> w117
            tunnel: w110 -> [w310]
            tunnel: [w310] -> w109
            frame #0 {
              # "DAQ Setup acquisition"
              n199 = local read "DAQ Number of Samples"() -> (w314:dbl)
              n200 = local read "DAQ Trigger Level (V)"() -> (w321:dbl)
              n201 = local read "DAQ Input Channel"() -> (w322:tag)
              n202 = local read "DAQ rate"() -> (w315:i32)
              n203 = call "RG Configure DAQ auto Max input scale.vi"("input terminal configuration"="DAQ Input Config", "DAQ Card Type"="DAQ Card", "Sampling rate"=w315, "DAQ Trigger Level"=w321, "physical channel"=w322, "number of samples"=w314) -> ("error out"=w313:errorcluster, "task out"=w312:refnum<k21>)  [unwired: 4 in]
              n204 = Reciprocal(x=w315) -> (1/x=w316:dbl)
              n205 = Initialize Array(0.0 ("element"), w314) -> (w317:dbl[])
              n206 = Bundle By Name("Y"=w317, "dt"=w316) -> (w311:waveform(dbl))  [unwired: 1 in]
            }
          }
          n207 = Max & Min(x=w106, y=700.0) -> (max(x,y)=w104:dbl)  [unwired: 1 out]
          n208 = local read "Trigger Level (V)"() -> (w280:dbl)
          n209 = local read "Trigger Source"() -> (w279:u16)
          n210 = local read "DAQ final number of points"() -> (w136:dbl)
          n211 = case shown="False" "Scope Channel Read" {
            tunnel: [w323 w327] -> w296
            tunnel: w285 -> [w324 w326]
            tunnel: w283 -> [_ w325]
            frame False {
              n212 = Build Array(w324) -> (w323:u16[])
            }
            frame True {
              n213 = Build Array(w326, w325) -> (w327:u16[])
            }
          }
          n214 = local read "Averages on scope"() -> (w201:i32)
          n215 = call "RG Configure Trigger (Edge).vi"("VISA resource name"=w277, "Trigger Source (0: Channel 1)"=w279, "Trigger Level (0.0 V)"=w280, "error in (no error)"=w276) -> ("VISA resource name out"=w272:refnum<visa-resource-name>, "error out"=w273:errorcluster)  [unwired: 10 in]
          n216 = local read "Final number of\nscope points"() -> (w266:dbl)
          n217 = call "Configure Acquisition.vi"("error in (no error)"=w273, "Number of Waveform Acquisitions (16)"=w201, "Acquisition Type (0: Sample)"="Acquisition Type", "VISA resource name"=w272) -> ("error out"=w101:errorcluster, "VISA resource name out"=w103:refnum<visa-resource-name>)  [unwired: 6 in]
          n218 = local write "Scope Error Counter"(w131) -> ()
          n219 = flat-sequence {
            tunnel: w103 -> [w309]
            tunnel: [w309] -> w102
            tunnel: w101 -> [w308]
            tunnel: [w308] -> w100
            frame #0 {
              n220 = Wait (ms)(milliseconds to wait=u32 1000) -> ()  [unwired: 1 out]
            }
          }
          n221 = Initialize Array(0.0 ("element"), w136) -> (w134:dbl[])
          n222 = Initialize Array(0.0 ("element"), w266) -> (w133:dbl[])
          n223 = while {
            tunnel: w296 -> [w345]
            tunnel: [w344] -> w163
            shift-right: [w356] -> w142
            shift-left: w100 -> [w349]
            shift-right: [w351] -> w143
            shift-left: w102 -> [w350]
            shift-right: [w381] -> w263
            shift-left: w133 -> [w364]
            shift-right: [w382] -> w297
            shift-left: w134 -> [w362]
            shift-right: [w358] -> w119
            shift-left: w131 -> [w363]
            shift-right: [w360] -> w264
            shift-left: w133 -> [w359]
            tunnel: 0 -> [w357]
            tunnel: w124 -> [w340]
            tunnel: w123 -> [w341]
            tunnel: [w339] -> w122
            tunnel: [w338] -> w121
            tunnel: w117 -> [w337]
            tunnel: w109 -> [_]
            tunnel: w104 -> [w328]
            stop <- w365 stop-if-true
            n224 = flat-sequence {
              tunnel: w350 -> [w438]
              tunnel: [w435] -> w346
              tunnel: [w434] -> w347
              tunnel: [w442] -> w336
              tunnel: w349 -> [w437]
              tunnel: w341 -> [w433]
              tunnel: w340 -> [w432]
              tunnel: [w431] -> w339
              tunnel: [w430] -> w338
              tunnel: w337 -> [w429]
              tunnel: w328 -> [w416]
              frame #0 {
                # "To synch DAQ and scope acquisitions"
                n225 = local read "Averages on scope"() -> (w441:i32)
                n226 = local read "DAQ LED line"() -> (w420:string)
                n227 = Equal?(x=w441, y=1.0) -> (x = y?=w439:bool)
                n228 = call "Initiate.vi"("error in (no error)"=w437, "VISA resource name"=w438) -> ("error out"=w426:errorcluster, "VISA resource name out"=w428:refnum<visa-resource-name>)  [unwired: 8 in]
                n229 = Multiply(x="LED on (s)", y=1000.0) -> (x*y=w421:dbl)
                n230 = case shown="True" w439 {
                  tunnel: [w482 w488] -> w442
                  tunnel: w433 -> [w481 w487]
                  tunnel: w432 -> [w480 w486]
                  tunnel: [w478 w485] -> w431
                  tunnel: [w477 w484] -> w430
                  tunnel: w429 -> [_ w483]
                  frame True {
                    # "No averages on scope, acquire one shot"
                    n231 = call-poly <vilib>:"DAQmx Read.vi"("task/channels in"=w481, "number of samples per channel"=-1, "timeout"=500.0, "error in"=w480) -> ("task out"=w478:refnum<k21>, "data"=w482:waveform(dbl), "error out"=w477:errorcluster)  [unwired: 9 in]
                  }
                  frame False {
                    # "Averaging on scope, acquire multiple shots."
                    n232 = while {
                      shift-right: [w502] -> w488
                      shift-left: w483 -> [w501]
                      tunnel: w487 -> [w495]
                      tunnel: w486 -> [w494]
                      tunnel: [w491] -> w485
                      tunnel: [w490] -> w484
                      i -> [w498]
                      stop <- w500 stop-if-true
                      n233 = call-poly <vilib>:"DAQmx Read.vi"("task/channels in"=w495, "number of samples per channel"=-1, "timeout"=20.0, "error in"=w494) -> ("task out"=w491:refnum<k21>, "data"=w496:waveform(dbl), "error out"=w490:errorcluster)  [unwired: 9 in]
                      n234 = local read "Averages on scope"() -> (w499:i32)
                      n235 = Add(x=w498, y=1) -> (x+y=w492:i32)
                      "DAQ Loop" <- w492
                      n236 = Greater Or Equal?(x=w492, y=w499) -> (x >= y?=w500:bool)
                      n237 = Add(1:w501, 2:w496) -> (0:w502:waveform(dbl))  [unwired: 1 in, 1 out]
                    }
                  }
                }
                n238 = Multiply(x="LED off (s)", y=1000.0) -> (x*y=w417:dbl)
                n239 = case shown="True" "PIA Mode" {
                  tunnel: w428 -> [w444 w458]
                  tunnel: [w444 w452] -> w427
                  tunnel: w426 -> [w443 w457]
                  tunnel: [w443 w453] -> w425
                  tunnel: w421 -> [_ w456]
                  tunnel: w420 -> [_ w451]
                  tunnel: w417 -> [_ w450]
                  tunnel: w416 -> [_ w445]
                  frame False {
                  }
                  frame True {
                    n240 = flat-sequence {
                      tunnel: w451 -> [w467]
                      tunnel: w457 -> [w468]
                      tunnel: w458 -> [w469]
                      tunnel: [w469] -> w449
                      tunnel: [w468] -> w448
                      tunnel: [w467] -> w447
                      tunnel: [w466] -> w446
                      tunnel: w445 -> [w465]
                      tunnel: [w474] -> w455
                      tunnel: [w475] -> w454
                      tunnel: [w473] -> _
                      tunnel: w456 -> [w472]
                      tunnel: w449 -> [w474]
                      tunnel: w448 -> [w475]
                      tunnel: w447 -> [w471]
                      tunnel: w446 -> [_]
                      frame #0 {
                        n241 = Wait (ms)(milliseconds to wait=w465) -> (millisecond timer value=w466:u32)
                      }
                      frame #1 {
                        n242 = call "RG DAQ control for PIA.vi"("lines"=w471, "Initial value"=TRUE) -> ()  [unwired: 10 in]
                        n243 = Wait (ms)(milliseconds to wait=w472) -> (millisecond timer value=w473:u32)
                      }
                    }
                    n244 = flat-sequence {
                      tunnel: w455 -> [w464]
                      tunnel: [w464] -> w452
                      tunnel: [w463] -> _
                      tunnel: w450 -> [w462]
                      tunnel: w451 -> [w461]
                      tunnel: w454 -> [w459]
                      tunnel: [w459] -> w453
                      frame #0 {
                        n245 = call "RG DAQ control for PIA.vi"("lines"=w461, "Initial value"=FALSE) -> ()  [unwired: 10 in]
                        n246 = Wait (ms)(milliseconds to wait=w462) -> (millisecond timer value=w463:u32)
                      }
                    }
                  }
                }
                n247 = VISA Write(VISA resource name=w427, write buffer="*WAI", error in (no error)=w425) -> (VISA resource name out=w435:refnum<visa-resource-name>, error out=w434:errorcluster)  [unwired: 1 out]
              }
            }
            n248 = local read "Scope Timeout (ms)"() -> (w348:u32)
            n249 = local read "DAQ Number of Samples"() -> (w332:dbl)
            n250 = call "RG Fetch Waveforms from scope.vi"("error in (no error)"=w347, "Maximum Time (10000ms)"=w348, "Channels"=w345, "VISA resource name"=w346) -> ("error out"=w342:errorcluster, "Waveform Data"=w344:waveform(dbl)[], "VISA resource name out"=w343:refnum<visa-resource-name>)  [unwired: 5 in]
            n251 = Unbundle By Name(w342) -> ("status"=w355:bool)
            n252 = local read "Scope average\nnumber of points"() -> (w378:dbl)
            n253 = local read "DAQ rate"() -> (w329:i32)
            n254 = Multiply(x=w332, y=-0.1) -> (x*y=w330:dbl)
            n255 = local read "DAQ average number of points"() -> (w369:dbl)
            n256 = Divide(x=w330, y=w329) -> (x/y=w333:dbl)
            n257 = Split Signals(w344) -> (w376:dynamicdata, w375:dynamicdata)  [unwired: 2 in]
            n258 = To Time Stamp(1:w333) -> (0:w335:timestamp)
            n259 = Unbundle By Name(w336) -> ("Y"=w370:dbl[])
            n260 = call "Convert from Dynamic Data2"("Dynamic Data Type"=w376) -> ("Array"=w354:dbl[])  [unwired: 3 in]
            n261 = call "Convert from Dynamic Data3"("Dynamic Data Type"=w375) -> ("Array"=w374:dbl[])  [unwired: 3 in]
            n262 = Empty Array?(array=w354) -> (empty?=w353:bool)
            n263 = Bundle By Name(cluster=w336, "t0"=w335) -> (→"DAQ Live Data":waveform(dbl))
            n264 = call-poly <vilib>:"Decimate (single shot).vi"("averaging"=TRUE, "decimating factor"=w369, "X"=w370) -> ("Decimated Array"=w361:dbl[])  [unwired: 7 in, 1 out]
            n265 = Not Or(1:w353, 2:w355) -> (0:w352:bool)
            n266 = call-poly <vilib>:"Decimate (single shot).vi"("averaging"=TRUE, "decimating factor"=w378, "X"=w354) -> ("Decimated Array"=w366:dbl[])  [unwired: 7 in, 1 out]
            n267 = call-poly <vilib>:"Decimate (single shot).vi"("averaging"=TRUE, "decimating factor"=w378, "X"=w374) -> ("Decimated Array"=w367:dbl[])  [unwired: 7 in, 1 out]
            n268 = case shown="False" w352 {
              tunnel: [w394 w415] -> w382
              tunnel: [w393 w414] -> w381
              tunnel: [w388 w405] -> w380
              tunnel: w367 -> [_ w413]
              tunnel: w366 -> [_ w412]
              tunnel: w364 -> [w393 w411]
              tunnel: w363 -> [w388 w410]
              tunnel: w362 -> [w394 w409]
              tunnel: w361 -> [_ w408]
              tunnel: [w392 w407] -> w360
              tunnel: w359 -> [w392 w406]
              tunnel: [w388 w405] -> w358
              tunnel: w357 -> [w390 _]
              tunnel: w342 -> [w386 w404]
              tunnel: [w384 w404] -> w356
              tunnel: w343 -> [w387 w403]
              tunnel: [w383 w403] -> w351
              frame False {
                # "Scope Error Detected"
                n269 = flat-sequence {
                  tunnel: w387 -> [w395]
                  tunnel: w386 -> [w396]
                  tunnel: [w395] -> w385
                  tunnel: w385 -> [w401]
                  tunnel: [w398] -> w384
                  tunnel: [w397] -> w383
                  frame #0 {
                    n270 = call "Close.vi"("error in (no error)"=w396, "VISA resource name"=w395) -> ()  [unwired: 9 in, 1 out]
                  }
                  frame #1 {
                    w400 = FALSE ("ID Query (True)")
                    n271 = call "Initialize.vi"("error in (no error)"=errorcluster {"status"=FALSE, "code"=0, "source"=""}, "Reset (True)"=w400, "ID Query (True)"=w400, "VISA resource name"=w401) -> ("error out"=w398:errorcluster, "VISA resource name out"=w397:refnum<visa-resource-name>)  [unwired: 6 in]
                  }
                }
                n272 = Add(x=w390, y=1.0) -> (x+y=→"Scope Error Counter":dbl)
              }
              frame True {
                # "No errors"
                n273 = local read "Averages on scope"() -> (w402:i32)
                n274 = Add(x=w402, y=w410) -> (x+y=w405:i32)
                "Readout Counter" <- w405
                n275 = Add(x=w408, y=w409) -> (x+y=w415:dbl[])
                n276 = Add(x=w411, y=w412) -> (x+y=w414:dbl[])
                n277 = Add(x=w413, y=w406) -> (x+y=w407:dbl[])
              }
            }
            n278 = local read "Number of Averages"() -> (w373:i32)
            n279 = Greater Or Equal?(x=w380, y=w373) -> (x >= y?=w372:bool)
            n280 = Or(x=w372, y="Stop Measurement") -> (x .or. y?=w365:bool)
          }
          n281 = call-poly <vilib>:"Index Waveform Array.vi"("index"=0, "waveform array"=w163) -> ("waveform"=w161:waveform(dbl))  [unwired: 8 in, 1 out]
          n282 = Unbundle By Name(w161) -> ("t0"=w141:timestamp, "dt"=w140:dbl)
          n283 = local read "Record Length"() -> (w157:u32)
          n284 = To Double Precision Float(number=w141) -> (double precision float=w160:dbl)
          n285 = local read "Scope average\nnumber of points"() -> (w154:dbl)
          n286 = Multiply(x=w157, y=1000.0) -> (x*y=w159:dbl)
          n287 = for {
            N: w159 -> [_]
            tunnel: w160 -> [w514]
            tunnel: w140 -> [w512]
            tunnel: [w510] -> w156 mode=indexing
            i -> [w513]
            n288 = Multiply(x=w512, y=w513) -> (x*y=w511:dbl)
            n289 = Add(x=w514, y=w511) -> (x+y=w510:dbl)
          }
          n290 = call-poly <vilib>:"Decimate (single shot).vi"("averaging"=TRUE, "decimating factor"=w154, "X"=w156) -> ("Decimated Array"=w153:dbl[])  [unwired: 7 in, 1 out]
          "Scope time axis" <- w153
          n291 = call <vilib>:"DAQmx Clear Task.vi"("task in"=w122, "error in"=w121) -> ()  [unwired: 13 in, 1 out]
          n292 = local read "Averages on scope"() -> (w120:i32)
          n293 = Divide(x=w119, y=w120) -> (x/y=w118:dbl)
          n294 = Divide(x=w264, y=w118) -> (x/y=w306:dbl[])
          n295 = Divide(x=w263, y=w118) -> (x/y=w197:dbl[])
          n296 = local read "DAQ final number of points"() -> (w116:dbl)
          n297 = Bundle By Name("Y"=w306, "t0"=w141, "dt"=w140) -> (→"Scope Average Channel2":waveform(dbl))  [unwired: 1 in]
          n298 = Bundle By Name("Y"=w197, "t0"=w141, "dt"=w140) -> (→"Scope Average Channel1":waveform(dbl))  [unwired: 1 in]
          n299 = local read "DAQ average number of points"() -> (w267:dbl)
          n300 = Divide(x=w297, y=w119) -> (x/y=w164:dbl[])
          n301 = local read "DAQ dt"() -> (w268:dbl)
          n302 = Multiply(x=w116, y=-0.1) -> (x*y=w113:dbl)
          n303 = Multiply(x=w268, y=w267) -> (x*y=w114:dbl)
          n304 = Multiply(x=w113, y=w114) -> (x*y=w111:dbl)
          n305 = To Time Stamp(1:w111) -> (0:w112:timestamp)
          n306 = local read "DAQ final number of points"() -> (w275:dbl)
          n307 = Bundle By Name("Y"=w164, "t0"=w112, "dt"=w114) -> (→"DAQ Average Data":waveform(dbl))  [unwired: 1 in]
          n308 = Multiply(x=w275, y=0.075) -> (x*y=w270:dbl)
          n309 = Round To Nearest(number=w270) -> (nearest integer value=w269:dbl)
          n310 = Array Subset(array=w164, index=0, length=w269) -> (w291:dbl[])
          n311 = local read "Amplification Factor"() -> (w289:dbl)
          n312 = Add Array Elements(numeric array=w291) -> (sum=w290:dbl)
          n313 = Divide(x=w290, y=w269) -> (x/y=w138:dbl)
          n314 = Multiply(x=w138, y=w289) -> (x*y=w139:dbl)
          n315 = local write "Background level (on Amp)"(w139) -> ()
          n316 = local write "Background level (V)"(w138) -> ()
          n317 = local read "DAQ Number of Samples"() -> (w145:dbl)
          n318 = for {
            N: w145 -> [_]
            tunnel: [w504] -> w146 mode=indexing
            i -> [w509]
            n319 = local read "DAQ Number of Samples"() -> (w508:dbl)
            n320 = Divide(x=w508, y=10.0) -> (x/y=w506:dbl)
            n321 = local read "DAQ dt"() -> (w503:dbl)
            n322 = Subtract(x=w509, y=w506) -> (x-y=w505:dbl)
            n323 = Multiply(x=w505, y=w503) -> (x*y=w504:dbl)
          }
          n324 = local read "DAQ average number of points"() -> (w148:dbl)
          n325 = Number To Decimal String(number=w176, width (-)=i16 3) -> (decimal integer string=w175:string)
          n326 = call-poly <vilib>:"Decimate (single shot).vi"("averaging"=TRUE, "decimating factor"=w148, "X"=w146) -> ("Decimated Array"=w144:dbl[])  [unwired: 7 in, 1 out]
          n327 = Concatenate Strings(w175, "nm Scope CH2 (raw data).txt") -> (w189:string)
          n328 = global read "global tas.vi" "Root Path"() -> (w255:path)
          n329 = Build Array(w144, w164) -> (w256:dbl[][])
          n330 = Build Array(w153, w197) -> (w246:dbl[][])
          n331 = global read "global tas.vi" "Root Path"() -> (w250:path)
          n332 = Concatenate Strings(w175, "nm DAQ (raw data).txt") -> (w192:string)
          n333 = global read "global tas.vi" "Root Path"() -> (w174:path)
          n334 = Build Array(w153, w306) -> (w251:dbl[][])
          n335 = Concatenate Strings(w175, "nm Scope CH1 (raw data).txt") -> (w187:string)
          n336 = Build Path(base path=w255, name or relative path=w192) -> (appended path=w254:path)
          n337 = Build Path(base path=w250, name or relative path=w189) -> (appended path=w249:path)
          n338 = Build Path(base path=w174, name or relative path=w187) -> (appended path=w245:path)
          n339 = call-poly <vilib>:"Write To Spreadsheet File.vi"("transpose? (no:F)"=TRUE, "format (%.3f)"="%.9f", "2D data"=w256, "file path (dialog if empty)"=w254) -> ()  [unwired: 4 in, 1 out]
          n340 = call-poly <vilib>:"Write To Spreadsheet File.vi"("transpose? (no:F)"=TRUE, "format (%.3f)"="%.9f", "2D data"=w246, "file path (dialog if empty)"=w245) -> ()  [unwired: 4 in, 1 out]
          n341 = call-poly <vilib>:"Write To Spreadsheet File.vi"("transpose? (no:F)"=TRUE, "format (%.3f)"="%.9f", "2D data"=w251, "file path (dialog if empty)"=w249) -> ()  [unwired: 4 in, 1 out]
          n342 = flat-sequence {
            tunnel: w175 -> [w648]
            tunnel: w174 -> [w647]
            tunnel: w137 -> [_]
            frame #0 {
              # "Write parameters file after values have been calculated."
              n343 = Build Array("Number of Averages", "Scope acq. type", "Number of averages on scope", "Scope average number of points", "Scope timebase (s)", "Scope CH1 vertical scale per div (V)", "Scope CH2 vertical scale per div (V)", "Background level on amp (V)", "DAQ sampling rate (Hz)", "DAQ average number of points", "Background level on DAQ (V)", "Amplification factor", "100% Reflection Reference Signal (V)" ("element"), "Output calculation Method" ("element")) -> (w672:string[])
              n344 = Concatenate Strings(w648, "nm Parameters.txt") -> (w650:string)
              n345 = local read "Averages on scope"() -> (w663:i32)
              n346 = local read "Scope Timebase"() -> (w664:dbl)
              n347 = local read "DAQ rate"() -> (w668:i32)
              n348 = local read "Acquisition Type"() -> (w681:u16)
              n349 = Build Path(base path=w647, name or relative path=w650) -> (appended path=w674:path)
              n350 = local read "Scope average\nnumber of points"() -> (w662:dbl)
              n351 = local read "Vertical Range CH TAS (10.0 V)"() -> (w665:dbl)
              n352 = local read "Vertical Range TPC (10.0 V)"() -> (w666:dbl)
              n353 = local read "Background level (on Amp)"() -> (w667:dbl)
              n354 = local read "DAQ average number of points"() -> (w669:dbl)
              n355 = local read "Background level (V)"() -> (w670:dbl)
              n356 = local read "Amplification Factor"() -> (w671:dbl)
              n357 = local read "100% Reflectance Standard (V)"() -> (w683:dbl)
              n358 = local read "Calculate Output Method"() -> (w685:T1)
              n359 = local read "Readout Counter"() -> (w679:i32)
              n360 = Build Array(w679, w681, w663, w662, w664, w665, w666, w667, w668, w669, w670, w671, w683, w685) -> (w673:dbl[])
              n361 = Number To Fractional String(number=w673) -> (F-format string=w649:string[])  [unwired: 3 in]
              n362 = Build Array(w672, w649) -> (w675:string[][])
              n363 = Array To Spreadsheet String(array=w675, 3:"%s" ("format string")) -> (spreadsheet string=w677:string)  [unwired: 1 in]
              n364 = Write to Text File(file (use dialog)=w674, text=w677) -> ()  [unwired: 2 in, 3 out]
            }
          }
          n365 = local read "Calculate Output Method"() -> (w209:T1)
          n366 = local read "TPC Multiplication factor"() -> (w230:dbl)
          n367 = case shown="\"Kubelka-Munk\"" w209 {
            tunnel: w164 -> [w716 w721 w739]
            tunnel: [w715 w719 w731] -> w229
            tunnel: w138 -> [w714 w718 w722]
            frame "Transmission" {
              # "Background level on DAQ"
              # "Calculate output as: deltaOD = log(T/T')"
              n368 = Divide(x=w714, y=w716) -> (x/y=w717:dbl[])
              n369 = Logarithm Base 10(1:w717) -> (0:w715:dbl[])
            }
            frame "Reflectance" {
              # "Calculate output as: Transient abs. = 1 - RT = (Rbkg - R(t)) / Rbkg"
              n370 = Subtract(x=w718, y=w721) -> (x-y=w720:dbl[])
              n371 = Divide(x=w720, y=w718) -> (x/y=w719:dbl[])
            }
            frame "Kubelka-Munk" {
              # "Calculate output from\nKM = (1-Rrelative)^2/(2*Rrelative)"
              n372 = local read "100% Reflectance Standard (V)"() -> (w738:dbl)
              n373 = Divide(x=w739, y=w738) -> (x/y=w724:dbl[])
              n374 = Subtract(x=1.0, y=w724) -> (x-y=w726:dbl[])
              n375 = Divide(x=w722, y=w738) -> (x/y=w733:dbl)
              n376 = Square(x=w726) -> (x^2=w727:dbl[])
              n377 = Subtract(x=1.0, y=w733) -> (x-y=w736:dbl)
              n378 = Multiply(x=w724, y=2.0) -> (x*y=w728:dbl[])
              n379 = Square(x=w736) -> (x^2=w735:dbl)
              n380 = Divide(x=w727, y=w728) -> (x/y=w723:dbl[])
              n381 = Multiply(x=w733, y=2.0) -> (x*y=w734:dbl)
              n382 = Divide(x=w735, y=w734) -> (x/y=w730:dbl)
              n383 = Subtract(x=w723, y=w730) -> (x-y=w731:dbl[])
            }
          }
          n384 = local read "DAQ average number of points"() -> (w202:dbl)
          n385 = local read "DAQ final number of points"() -> (w213:dbl)
          n386 = Multiply(x=w306, y=w230) -> (x*y=w237:dbl[])
          n387 = local read "DAQ dt"() -> (w203:dbl)
          n388 = local read "Scope pretrigger points"() -> (w217:dbl)
          n389 = Multiply(x=w203, y=w202) -> (x*y=w204:dbl)
          n390 = Divide(x=w213, y=-10.0) -> (x/y=w212:dbl)
          n391 = Multiply(x=w212, y=w204) -> (x*y=w211:dbl)
          n392 = To Time Stamp(1:w211) -> (0:w210:timestamp)
          n393 = Multiply(x=w217, y=0.75) -> (x*y=w216:dbl)
          n394 = Bundle By Name("Y"=w237, "t0"=w141, "dt"=w140) -> (→"Scope CH2 data (final)":waveform(dbl))  [unwired: 1 in]
          n395 = Array Subset(array=w197, index=0, length=w216) -> (w220:dbl[])
          n396 = Add Array Elements(numeric array=w220) -> (sum=w221:dbl)
          n397 = Divide(x=w221, y=w216) -> (x/y=w222:dbl)
          n398 = Subtract(x=w197, y=w222) -> (x-y=w208:dbl[])
          n399 = local read "Calculate Output Method"() -> (w205:T1)
          n400 = Bundle By Name("Y"=w229, "t0"=w210, "dt"=w204) -> (→"DAQ DOD data (final)":waveform(dbl))  [unwired: 1 in]
          n401 = Add(x=w208, y=w139) -> (x+y=w207:dbl[])
          n402 = case shown="\"Reflectance\"" w205 {
            tunnel: w207 -> [w687 w693 w712]
            tunnel: [w686 w690 w705] -> w206
            frame "Transmission" {
              # "Calculate output as: deltaOD = log(T/T')"
              n403 = local read "Background level (on Amp)"() -> (w688:dbl)
              n404 = Divide(x=w688, y=w687) -> (x/y=w689:dbl[])
              n405 = Logarithm Base 10(1:w689) -> (0:w686:dbl[])
            }
            frame "Reflectance" {
              # "Calculate output as: Transient abs. = 1 - RT = (Rbkg - R(t)) / Rbkg"
              n406 = local read "Background level (on Amp)"() -> (w692:dbl)
              n407 = Subtract(x=w692, y=w693) -> (x-y=w691:dbl[])
              n408 = Divide(x=w691, y=w692) -> (x/y=w690:dbl[])
            }
            frame "Kubelka-Munk" {
              # "Calculate output from\nKM = (1-Rrelative)^2/(2*Rrelative)"
              n409 = local read "100% Reflectance Standard (V)"() -> (w695:dbl)
              n410 = local read "Amplification Factor"() -> (w696:dbl)
              n411 = local read "Background level (on Amp)"() -> (w713:dbl)
              n412 = Multiply(x=w695, y=w696) -> (x*y=w694:dbl)
              n413 = Divide(x=w712, y=w694) -> (x/y=w698:dbl[])
              n414 = Subtract(x=1.0, y=w698) -> (x-y=w700:dbl[])
              n415 = Divide(x=w713, y=w694) -> (x/y=w707:dbl)
              n416 = Square(x=w700) -> (x^2=w701:dbl[])
              n417 = Subtract(x=1.0, y=w707) -> (x-y=w710:dbl)
              n418 = Multiply(x=w698, y=2.0) -> (x*y=w702:dbl[])
              n419 = Square(x=w710) -> (x^2=w709:dbl)
              n420 = Divide(x=w701, y=w702) -> (x/y=w697:dbl[])
              n421 = Multiply(x=w707, y=2.0) -> (x*y=w708:dbl)
              n422 = Divide(x=w709, y=w708) -> (x/y=w704:dbl)
              n423 = Subtract(x=w697, y=w704) -> (x-y=w705:dbl[])
            }
          }
          n424 = local read "DAQ Number of Samples"() -> (w218:dbl)
          n425 = for {
            N: w218 -> [_]
            tunnel: [w741] -> w152 mode=indexing
            i -> [w746]
            n426 = local read "DAQ Number of Samples"() -> (w745:dbl)
            n427 = Divide(x=w745, y=10.0) -> (x/y=w743:dbl)
            n428 = local read "DAQ dt"() -> (w740:dbl)
            n429 = Subtract(x=w746, y=w743) -> (x-y=w742:dbl)
            n430 = Multiply(x=w742, y=w740) -> (x*y=w741:dbl)
          }
          n431 = Number To Decimal String(number=w176, width (-)=i16 3) -> (decimal integer string=w178:string)
          n432 = local read "DAQ average number of points"() -> (w149:dbl)
          n433 = Concatenate Strings(w178, "nm Scope CH1 (final A).txt") -> (w180:string)
          n434 = Build Array(w153, w237) -> (w236:dbl[][])
          n435 = global read "global tas.vi" "Root Path"() -> (w226:path)
          n436 = Concatenate Strings(w178, "nm Scope CH2 (final).txt") -> (w182:string)
          n437 = global read "global tas.vi" "Root Path"() -> (w235:path)
          n438 = Build Path(base path=w226, name or relative path=w180) -> (appended path=w225:path)
          n439 = Build Path(base path=w235, name or relative path=w182) -> (appended path=w234:path)
          n440 = call-poly <vilib>:"Decimate (single shot).vi"("averaging"=TRUE, "decimating factor"=w149, "X"=w152) -> ("Decimated Array"=w151:dbl[])  [unwired: 7 in, 1 out]
          n441 = call-poly <vilib>:"Write To Spreadsheet File.vi"("transpose? (no:F)"=TRUE, "format (%.3f)"="%.9f", "2D data"=w236, "file path (dialog if empty)"=w234) -> ()  [unwired: 4 in, 1 out]
          n442 = Bundle By Name("Y"=w206, "t0"=w141, "dt"=w140) -> (w199:waveform(dbl))  [unwired: 1 in]
          "Scope CH1 DOD data (A final)" <- w199
          n443 = Build Array(w151, w229) -> (w228:dbl[][])
          n444 = global read "global tas.vi" "Root Path"() -> (w239:path)
          n445 = Build Array(w153, w206) -> (w227:dbl[][])
          n446 = call-poly <vilib>:"Write To Spreadsheet File.vi"("transpose? (no:F)"=TRUE, "format (%.3f)"="%.9f", "2D data"=w227, "file path (dialog if empty)"=w225) -> ("new file path (Not A Path if cancelled)"=w137:path)  [unwired: 4 in]
          n447 = Concatenate Strings(w178, "nm DAQ DOD (final).txt") -> (w184:string)
          n448 = local read "Trace B ?"() -> (w200:bool)
          n449 = Build Path(base path=w239, name or relative path=w184) -> (appended path=w240:path)
          n450 = case shown="True" w200 {
            tunnel: w199 -> [_ _]
            tunnel: [u32 0 ("millisecond timer value") w870] -> w198
            tunnel: w119 -> [_ _]
            frame False {
            }
            frame True {
              w883 = u32 10000  # timeout (10sec)
              # "Note:Closing the serial port allows it to be used by other applications without quitting LabVIEW."
              # "Close session to port."
              # "Configure Serial port (baud rate, data bits, parity, stop bits and flow control)."
              # "Write bytes to port."
              n451 = Wait (ms)(milliseconds to wait=u32 20000) -> (millisecond timer value=w870:u32)
              n452 = local read "Shutter VISA resource name"() -> (w877:refnum<visa-resource-name>)
              n453 = local read "Shutter data bits"() -> (w874:u16)
              n454 = local read "Shutter baud rate"() -> (w876:u32)
              n455 = local read "Shutter parity"() -> (w875:u16)
              n456 = local read "Shutter flow control"() -> (w873:u16)
              n457 = local read "Shutter stop bits"() -> (w872:u16)
              n458 = local read "Shutter open string"() -> (w869:string)
              n459 = call-poly "VISA Configure Serial Port"("VISA resource name"=w877, "timeout (10sec)"=w883, "baud rate (9600)"=w876, "data bits (8)"=w874, "parity (0:none)"=w875, "stop bits (10: 1 bit)"=w872, "flow control (0:none)"=w873) -> ("VISA resource name out"=w882:refnum<visa-resource-name>, "error out"=w881:errorcluster)  [unwired: 2 in, 5 out]
              n460 = VISA Write(VISA resource name=w882, write buffer=w869, error in (no error)=w881) -> (VISA resource name out=w879:refnum<visa-resource-name>, error out=w878:errorcluster)  [unwired: 1 out]
              n461 = VISA Close(VISA resource name=w879, error in (no error)=w878) -> (error out=w880:errorcluster)
              n462 = call <vilib>:"Simple Error Handler.vi"("error in (no error)"=w880) -> ()  [unwired: 1 in, 8 out]
            }
          }
          n463 = call-poly <vilib>:"Write To Spreadsheet File.vi"("transpose? (no:F)"=TRUE, "format (%.3f)"="%.9f", "2D data"=w228, "file path (dialog if empty)"=w240) -> ()  [unwired: 4 in, 1 out]
          n464 = case shown="True" w200 {
            tunnel: w208 -> [_ w800]
            tunnel: w198 -> [_ _]
            tunnel: [w750 w759] -> w177
            tunnel: w176 -> [_ w758]
            tunnel: w153 -> [_ w757]
            tunnel: w143 -> [w748 w756]
            tunnel: w142 -> [w747 w755]
            frame False {
              n465 = call "Close.vi"("error in (no error)"=w747, "VISA resource name"=w748) -> ("error out"=w749:errorcluster)  [unwired: 9 in]
              n466 = call <vilib>:"Simple Error Handler.vi"("error in (no error)"=w749) -> ()  [unwired: 4 in, 5 out]
              n467 = Wait (ms)(milliseconds to wait=u32 1) -> (millisecond timer value=w750:u32)
            }
            frame True {
              # "Scope time axis"
              # "Current wavelength"
              n468 = local read "Final number of\nscope points"() -> (w772:dbl)
              n469 = Initialize Array(0.0 ("element"), w772) -> (w773:dbl[])
              n470 = while {
                tunnel: w756 -> [w810]
                tunnel: [w819] -> w807
                tunnel: w755 -> [w809]
                tunnel: [w818] -> w808
                shift-right: [w837] -> w775
                shift-left: w773 -> [w836]
                shift-right: [w820] -> w754
                shift-left: 0 -> [w821]
                stop <- w833 stop-if-true
                n471 = local read "Channel TAS (0: Channel 1)"() -> (w815:u16)
                n472 = local read "Scope Timeout (ms)"() -> (w816:u32)
                n473 = call "RG Read (Single Waveform) change OPC for WAIT.vi"("error in (no error)"=w809, "Maximum Time (10000ms)"=w816, "Channel (0: Channel 1)"=w815, "VISA resource name"=w810) -> ("error out"=w812:errorcluster, "Waveform Graph"=w814:waveform(dbl), "VISA resource name out"=w813:refnum<visa-resource-name>)  [unwired: 5 in]
                "B trace (Channel1)" <- w814
                n474 = local read "Scope average\nnumber of points"() -> (w838:dbl)
                n475 = Unbundle By Name(w814) -> ("Y"=w831:dbl[])
                n476 = local read "Final number of\nscope points"() -> (w830:dbl)
                n477 = local read "Averages on scope"() -> (w811:i32)
                n478 = call-poly <vilib>:"Decimate (single shot).vi"("averaging"=TRUE, "decimating factor"=w838, "X"=w831) -> ("Decimated Array"=w827:dbl[])  [unwired: 7 in, 1 out]
                n479 = Array Size(array=w827) -> (size(s)=w826:i32)
                n480 = Initialize Array(0.0 ("element"), w830) -> (w828:dbl[])
                n481 = Equal To 0?(x=w826) -> (x = 0?=w823:bool)
                n482 = Select(t=0.0, s=w823, f=w811) -> (s? t:f=w822:dbl)
                n483 = Add(x=w821, y=w822) -> (x+y=w820:dbl)
                "Btrace Readout Counter" <- w820
                n484 = local read "Number of Averages"() -> (w835:i32)
                n485 = Select(t=w828, s=w823, f=w827) -> (s? t:f=w825:dbl[])
                n486 = VISA Write(VISA resource name=w813, write buffer="*WAI", error in (no error)=w812) -> (VISA resource name out=w819:refnum<visa-resource-name>, error out=w818:errorcluster)  [unwired: 1 out]
                n487 = Add(x=w836, y=w825) -> (x+y=w837:dbl[])
                n488 = Greater Or Equal?(x=w820, y=w835) -> (x >= y?=w834:bool)
                n489 = Or(x=w834, y="Stop Btrace Measurement") -> (x .or. y?=w833:bool)
              }
              n490 = Number To Decimal String(number=w758, width (-)=i16 3) -> (decimal integer string=w761:string)
              n491 = Concatenate Strings(w761, "nm Scope CH1 B trace (raw data).txt") -> (w765:string)
              n492 = global read "global tas.vi" "Root Path"() -> (w777:path)
              n493 = Build Path(base path=w777, name or relative path=w765) -> (appended path=w776:path)
              n494 = local read "Averages on scope"() -> (w753:i32)
              n495 = Divide(x=w754, y=w753) -> (x/y=w752:dbl)
              n496 = local read "Scope pretrigger points"() -> (w784:dbl)
              n497 = Divide(x=w775, y=w752) -> (x/y=w774:dbl[])
              n498 = call "Close.vi"("error in (no error)"=w808, "VISA resource name"=w807) -> ("error out"=w806:errorcluster)  [unwired: 9 in]
              n499 = Build Array(w757, w774) -> (w780:dbl[][])
              n500 = call <vilib>:"Simple Error Handler.vi"("error in (no error)"=w806) -> ()  [unwired: 4 in, 5 out]
              n501 = call-poly <vilib>:"Write To Spreadsheet File.vi"("transpose? (no:F)"=TRUE, "format (%.3f)"="%.9f", "2D data"=w780, "file path (dialog if empty)"=w776) -> ()  [unwired: 4 in, 1 out]
              n502 = Multiply(x=w784, y=0.75) -> (x*y=w785:dbl)
              n503 = Array Subset(array=w774, index=0, length=w785) -> (w803:dbl[])
              n504 = Add Array Elements(numeric array=w803) -> (sum=w804:dbl)
              n505 = Divide(x=w804, y=w785) -> (x/y=w805:dbl)
              n506 = local read "Background level (on Amp)"() -> (w769:dbl)
              n507 = Subtract(x=w774, y=w805) -> (x-y=w801:dbl[])
              n508 = local read "Calculate Output Method"() -> (w781:T1)
              n509 = Subtract(x=w800, y=w801) -> (x-y=w770:dbl[])
              n510 = Add(x=w770, y=w769) -> (x+y=w771:dbl[])
              n511 = case shown="\"Reflectance\"" w781 {
                tunnel: w771 -> [w841 w847 w866]
                tunnel: [w840 w844 w859] -> w782
                frame "Transmission" {
                  # "Calculate output as: deltaOD = log(T/T')"
                  n512 = local read "Background level (on Amp)"() -> (w842:dbl)
                  n513 = Divide(x=w842, y=w841) -> (x/y=w843:dbl[])
                  n514 = Logarithm Base 10(1:w843) -> (0:w840:dbl[])
                }
                frame "Reflectance" {
                  # "Calculate output as: Transient abs. = 1 - RT = (Rbkg - R(t)) / Rbkg"
                  n515 = local read "Background level (on Amp)"() -> (w846:dbl)
                  n516 = Subtract(x=w846, y=w847) -> (x-y=w845:dbl[])
                  n517 = Divide(x=w845, y=w846) -> (x/y=w844:dbl[])
                }
                frame "Kubelka-Munk" {
                  # "Calculate output from\nKM = (1-Rrelative)^2/(2*Rrelative)"
                  n518 = local read "100% Reflectance Standard (V)"() -> (w849:dbl)
                  n519 = local read "Amplification Factor"() -> (w850:dbl)
                  n520 = local read "Background level (on Amp)"() -> (w867:dbl)
                  n521 = Multiply(x=w849, y=w850) -> (x*y=w848:dbl)
                  n522 = Divide(x=w866, y=w848) -> (x/y=w852:dbl[])
                  n523 = Subtract(x=1.0, y=w852) -> (x-y=w854:dbl[])
                  n524 = Divide(x=w867, y=w848) -> (x/y=w861:dbl)
                  n525 = Square(x=w854) -> (x^2=w855:dbl[])
                  n526 = Subtract(x=1.0, y=w861) -> (x-y=w864:dbl)
                  n527 = Multiply(x=w852, y=2.0) -> (x*y=w856:dbl[])
                  n528 = Square(x=w864) -> (x^2=w863:dbl)
                  n529 = Divide(x=w855, y=w856) -> (x/y=w851:dbl[])
                  n530 = Multiply(x=w861, y=2.0) -> (x*y=w862:dbl)
                  n531 = Divide(x=w863, y=w862) -> (x/y=w858:dbl)
                  n532 = Subtract(x=w851, y=w858) -> (x-y=w859:dbl[])
                }
              }
              n533 = local read "Scope pretrigger points"() -> (w786:dbl)
              n534 = local read "Scope Timebase"() -> (w787:dbl)
              n535 = Divide(x=w787, y=10.0) -> (x/y=w793:dbl)
              n536 = Divide(x=w787, y=w786) -> (x/y=w788:dbl)
              n537 = Multiply(x=w793, y=-1.0) -> (x*y=w790:dbl)
              n538 = To Time Stamp(1:w790) -> (0:w789:timestamp)
              n539 = global read "global tas.vi" "Root Path"() -> (w795:path)
              n540 = Bundle By Name("Y"=w782, "t0"=w789, "dt"=w788) -> (→"Scope CH1 DOD data (A-B final)":waveform(dbl))  [unwired: 1 in]
              n541 = Concatenate Strings(w761, "nm Scope CH1 (final A-B).txt") -> (w763:string)
              n542 = Build Path(base path=w795, name or relative path=w763) -> (appended path=w796:path)
              n543 = Wait (ms)(milliseconds to wait=u32 1) -> (millisecond timer value=w759:u32)
              n544 = Build Array(w757, w782) -> (w794:dbl[][])
              n545 = call-poly <vilib>:"Write To Spreadsheet File.vi"("transpose? (no:F)"=TRUE, "format (%.3f)"="%.9f", "2D data"=w794, "file path (dialog if empty)"=w796) -> ()  [unwired: 4 in, 1 out]
            }
          }
        }
        n546 = flat-sequence {
          tunnel: w61 -> [_]
          frame #0 {
            w94 = FALSE
            n547 = local write "2b - Spectrum"(w94) -> ()
            n548 = local write "2a - Kinetic"(w94) -> ()
            n549 = One Button Dialog(message="Acquisition complete.") -> ()  [unwired: 1 in, 1 out]
          }
        }
      }
      frame 3 {
        # "Code"
        n550 = case shown="False" w966 {
          tunnel: w966 -> [w1043 w1057]
          tunnel: [w1040 w1057] -> w965
          frame False {
            # "PTI Mono"
            n551 = flat-sequence {
              tunnel: [w1050] -> w1044
              tunnel: w1043 -> [w1050]
              tunnel: w1044 -> [w1056]
              tunnel: [w1056] -> w1041
              tunnel: [w1052] -> w1042
              frame #0 {
                # "Check where mono is"
                n552 = call "UserInputMonoValue.vi"() -> ("Monochromator readout"=w1051:dbl)  [unwired: 17 in, 2 out]
                n553 = local write "Current Wavelength (PTI)"(w1051) -> ()
              }
              frame #1 {
                # "Find out which grating is currently being used"
                n554 = Two Button Dialog(message="Please press the appropriate\nbutton for the grating currently\nselected on the monochromator.", 1:"Visible" ("F button name (\"Cancel\")"), 2:"IR" ("T button name (\"OK\")")) -> (T button?=w1052:bool)
                n555 = local write "Is IR"(w1052) -> ()
              }
            }
            n556 = case shown="True" w1042 {
              tunnel: w1041 -> [w1045 w1046]
              tunnel: [w1045 w1046] -> w1040
              frame False {
              }
              frame True {
                n557 = local read "Current Wavelength (PTI)"() -> (w1049:dbl)
                n558 = Multiply(x=w1049, y=2.0) -> (x*y=w1048:dbl)
                n559 = local write "Current Wavelength (PTI)"(w1048) -> ()
              }
            }
          }
          frame True {
            # "Oriel Mono"
          }
        }
        n560 = case shown="True" w965 {
          tunnel: [w968 w1028] -> w967
          frame False {
            # "PTI Mono"
            n561 = flat-sequence {
              tunnel: [w972] -> w969
              tunnel: [w1022] -> _
              tunnel: w969 -> [w1022]
              tunnel: [w1021] -> w968
              frame #0 {
                n562 = local read "Is IR"() -> (w971:bool)
                n563 = call "RG Get User Input Wavelength.vi"() -> ("Go to wavelength"=w970:i32)  [unwired: 11 in]
                n564 = case shown="True" w971 {
                  tunnel: [w975 w998] -> w972
                  tunnel: w970 -> [w974 w997]
                  tunnel: w970 -> [w973 w996]
                  frame True {
                    # "Currently in IR"
                    n565 = Greater?(x=w973, y=1000.0) -> (0:w976:bool)
                    n566 = case shown="True" w976 {
                      tunnel: [w979 w988] -> w975
                      tunnel: w974 -> [w978 w987]
                      frame False {
                        n567 = stacked-sequence {
                          seq-local: [_ w984 _] -> [_ _ w986]
                          tunnel: [_ _ w986] -> w979
                          tunnel: w978 -> [_ w984 _]
                          frame #0 {
                            # "switch to visible\nand recal mono"
                            n568 = One Button Dialog(message="Please switch\nto the visible grating\nnow.") -> (true=w980:bool)  [unwired: 1 in]
                            n569 = case shown="True" w980 {
                              frame False {
                              }
                              frame True {
                                n570 = call "UserInputMonoValue.vi"() -> ("Monochromator readout"=w982:dbl)  [unwired: 17 in, 2 out]
                                n571 = local write "Is IR"(FALSE ("Is IR")) -> ()
                                n572 = local write "Current Wavelength (PTI)"(w982) -> ()
                              }
                            }
                          }
                          frame #1 {
                            # "now in visible, move \nto new wavelength"
                            n573 = local read "Current Wavelength (PTI)"() -> (w985:dbl)
                            n574 = call "ChazMoveMono.vi"("Move to"=w984, "Current"=w985) -> ()  [unwired: 8 in, 2 out]
                          }
                          frame #2 {
                            n575 = local write "Current Wavelength (PTI)"(w986) -> ()
                          }
                        }
                      }
                      frame True {
                        # "Still in IR"
                        n576 = stacked-sequence {
                          seq-local: [w989 _] -> [_ w995]
                          tunnel: [_ w995] -> w988
                          tunnel: w987 -> [w989 _]
                          frame #0 {
                            n577 = local read "Current Wavelength (PTI)"() -> (w994:dbl)
                            n578 = Divide(x=w989, y=2.0) -> (x/y=w990:dbl)
                            n579 = Divide(x=w994, y=2.0) -> (x/y=w991:dbl)
                            n580 = call "ChazMoveMono.vi"("Move to"=w990, "Current"=w991) -> ()  [unwired: 8 in, 2 out]
                          }
                          frame #1 {
                            n581 = local write "Current Wavelength (PTI)"(w995) -> ()
                          }
                        }
                      }
                    }
                  }
                  frame False {
                    # "Currently in Visible"
                    n582 = Greater?(x=w996, y=1000.0) -> (0:w999:bool)
                    n583 = case shown="True" w999 {
                      tunnel: [w1002 w1007] -> w998
                      tunnel: w997 -> [w1001 w1006]
                      frame False {
                        # "Still in Visible"
                        n584 = stacked-sequence {
                          seq-local: [w1003 _] -> [_ w1005]
                          tunnel: [_ w1005] -> w1002
                          tunnel: w1001 -> [w1003 _]
                          frame #0 {
                            n585 = local read "Current Wavelength (PTI)"() -> (w1004:dbl)
                            n586 = call "ChazMoveMono.vi"("Move to"=w1003, "Current"=w1004) -> ()  [unwired: 8 in, 2 out]
                          }
                          frame #1 {
                            n587 = local write "Current Wavelength (PTI)"(w1005) -> ()
                          }
                        }
                      }
                      frame True {
                        n588 = stacked-sequence {
                          seq-local: [_ w1014 _] -> [_ _ w1020]
                          tunnel: [_ _ w1020] -> w1007
                          tunnel: w1006 -> [_ w1014 _]
                          frame #0 {
                            # "switch to IR\nand recal mono"
                            n589 = One Button Dialog(message="Please switch\nto the IR grating\nnow.") -> (true=w1008:bool)  [unwired: 1 in]
                            n590 = case shown="True" w1008 {
                              frame False {
                              }
                              frame True {
                                n591 = call "UserInputMonoValue.vi"() -> ("Monochromator readout"=w1012:dbl)  [unwired: 17 in, 2 out]
                                n592 = local write "Is IR"(TRUE ("Is IR")) -> ()
                                n593 = Multiply(x=w1012, y=2.0) -> (x*y=w1010:dbl)
                                n594 = local write "Current Wavelength (PTI)"(w1010) -> ()
                              }
                            }
                          }
                          frame #1 {
                            # "now in IR, move \nto new wavelength"
                            n595 = local read "Current Wavelength (PTI)"() -> (w1017:dbl)
                            n596 = Divide(x=w1014, y=2.0) -> (x/y=w1015:dbl)
                            n597 = Divide(x=w1017, y=2.0) -> (x/y=w1016:dbl)
                            n598 = call "ChazMoveMono.vi"("Move to"=w1015, "Current"=w1016) -> ()  [unwired: 8 in, 2 out]
                          }
                          frame #2 {
                            n599 = local write "Current Wavelength (PTI)"(w1020) -> ()
                          }
                        }
                      }
                    }
                  }
                }
              }
              frame #1 {
                n600 = call <vilib>:"General Error Handler.vi"() -> ("error out"=w1021:errorcluster)  [unwired: 11 in, 4 out]
              }
            }
          }
          frame True {
            # "Oriel Mono"
            n601 = call "m_open.vi"() -> ("error out"=w1038:errorcluster, "configuration file path copy"=w1039:path)  [unwired: 2 in]
            n602 = call "GetWave.vi"("error in (no error)"=w1038) -> ("error out"=w1031:errorcluster, "Present Wavelength"=w1027:dbl)  [unwired: 1 in]
            n603 = call "RG Get User Input Wavelength.vi"("Current wavelength"=w1027) -> ("Go to wavelength"=w1026:i32)  [unwired: 10 in]
            n604 = call "getgrat.vi"("error in (no error)"=w1031) -> ("error out"=w1032:errorcluster, "Grating"=→"Grating":i32)  [unwired: 1 in]
            n605 = Less Or Equal?(x=w1026, y=590.0) -> (x <= y?=w1029:bool)
            n606 = Select(t=1.0, s=w1029, f=2.0) -> (s? t:f=w1033:dbl)
            n607 = call "setgrat.vi"("error in (no error)"=w1032, "Grating"=w1033) -> ("error out"=w1030:errorcluster)  [unwired: 1 in]
            n608 = call "gowave.vi"("error in (no error)"=w1030, "Destination Wavelength"=w1026) -> ("error out"=w1025:errorcluster)
            n609 = call "GetWave.vi"("error in (no error)"=w1025) -> ("error out"=w1024:errorcluster, "Present Wavelength"=w1023:dbl)  [unwired: 1 in]
            n610 = local write "Current wavelength (Oriel)"(w1023) -> ()
            n611 = call "m_close.vi"("error in (no error)"=w1024, "configuration file path"=w1039) -> ("error out"=w1028:errorcluster)  [unwired: 1 out]
          }
        }
        n612 = flat-sequence {
          tunnel: w967 -> [_]
          frame #0 {
            n613 = local write "3 - Move mono"(FALSE ("3 - Move shutter")) -> ()
            n614 = One Button Dialog(message="Wavelength change complete.") -> ()  [unwired: 1 in, 1 out]
          }
        }
      }
    }
  }
